vi "Save File DOE File Setup.vi"(0 "Filepath In":T10, 2 "Washer Controls In":T12={"Test Fixture Hardware"={"Power "={"Yokogawa"={"WT210"={"Sample Rate (1: 0.25s)"=1, "A Range (12: 20A)"=12, "V Range (6: 600V)"=4, "Power VISA Yokogawa WT210"="WT210"}, "WT500"={"Power VISA Yokogawa WT500"="WT500", "V Range (8: 1000V)"=0, "I Range (7: 40A)"=0, "Update Rate (3: 500ms)"=2}, "WT310_2"={"Sample Rate (1: 0.25s)"=1, "A Range (12: 20A)"=11, "V Range (6: 600V)"=4, "Power VISA Yokogawa WT310_2"="WT310_2"}, "WT310_3"={"Sample Rate (1: 0.25s)"=1, "A Range (12: 20A)"=11, "V Range (6: 600V)"=4, "Power VISA Yokogawa WT310_3"="WT310_3"}}, "Aplus"={"Aplus IP Address"="192.168.1.101", "Remote Port"=502, "Instrument"="APLUS", "Instr Driver Revision"="1.03.0053"}, "Power Limits"={"Crest Factor"={"Upper Limit"=1.49, "Lower Limit"=1.34}, "Harmonic Content"={"Uthd"=2.0}, "Voltage"={"% Error"=2.0}, "Stability"={"<1 Watt "={"Wattage"=1.0, "Slope (mW/H)"=10.0}, ">1 Watt"={"1%Power/Hour"=1.0}}}, "Nominal Voltage"=120, "Time Limit (s)"=10800.0, "Power Variation Limit (%)"=50.0, "Power Supply"={"Chroma 61605"="CHROMA", "Use Chroma?"=FALSE}}, "Weight Scale"={"Com Options"={"IND560Scale VISA"="IND560", "IP Address"="192.168.1.50", "Remote Port"=502, "Setra Scale VISA"="MW100", "GSE 350"="GSE350"}, "Select Scale"=""}, "Flow Rates"={"Laurel Cold IP Address"="", "Laurel Hot IP Address"="34972A_2", "Hot Water Laurel VISA"="LaurelMeter_Hot", "Cold Water Laurel VISA"="LaurelMeter_Cold", "Remote Port"=0, "Laurel Communication Type"="", "Meters To Collect (Hot Cold)"="", "HOT Laurel Reference"=refnum, "COLD Laurel Reference"=refnum}, "Analog Data"={"Agilent"={"Agilent 34972_1"="34972A_1", "Agilent 34972_2"="34972A_2", "Agilent 34972_3"="34972A_3", "Agilent 34972_4"="34972A_4", "Agilent 34972_5"="34972A_5", "Agilent 34972_6"="34972A_6", "Agilent Gain"=0.0, "TC Type (K,J,T)"="", "Instrument IDN?"="", "TC Channels-List"="", "Analog Channels-List"="", "Agilent Cluster Array"=[], "TC Channels-List 2"="", "Analog Channels-List 2"=""}, "Yokogawa"={"MW100"="MW100", "Intellifaucet"=FALSE}, "Select Analog"="", "TC Coefficients"={"TC Coefficients 1"=[], "TC Coefficients 2"=[], "TC Coefficients 3"=[], "TC Coefficients 4"=[], "TC Coefficients 5"=[], "TC Coefficients 6"=[], "TC Coefficients 7"=[]}, "NI Tasks (Dryer DOE)"=["TC Temps-Module 1", "TC Temps-Module 2", "TC Temps-Module 3", "TC Temps-Module 4", "TC Temps-Module 5", "Gas and Temp-Module 6", "AC_DC Events-Module 7"], "Laurel Analog"={"Laurel IP (Water Temp)"="", "Laurel IP (Pressure)"=""}}, "ITHX-Temp Humidity"={"IP Address 1"="", "Remote Port"=0, "IP Address 2"="", "IP Address 3"=""}, "Gas Meter COM Ports"={"Gas Meter 1"="COM3", "Gas Meter 2"="COM4", "Gas Meter 3"="COM5", "Gas Meter 4"="COM6", "Gas Meter 5"="COM7", "Gas Meter 6"="COM8"}, "Barometric Pressure"={"HEISE 901A"="HEISE", "Use Barometer?"=FALSE}}, "GEA2"={"Address"=35, "Source"=228, "Viper/Hawk"=0}, "DOE Capacity Measurments"={"Weight 1"=35.0, "Model Number 1"="", "Temp 1"=0.0, "Serial Number 1"="", "Lab Number 1"="", "Lab Number 2"="", "Serial Number 2"="", "Temp 2"=0.0, "Model Number 2"="", "Weight 2"=0.0, "Lab Number 3"="", "Serial Number 3"="", "Temp 3"=0.0, "Model Number 3"="", "Weight 3"=0.0, "Lab Number 4"="", "Serial Number 4"="", "Temp 4"=0.0, "Model Number 4"="", "Weight 4"=0.0, "Capacity Measurment Output String"=[]}, "Initialize.Washer In"={"Appliance Details"={"FileVersionInfo"={"FileVersion"="", "ProductName"="", "InternalName"="", "CompanyName"="", "LegalCopyright"="", "FileDescription"=""}, "Dishwasher Info"={"Open Cup Weight (gm):"=0.0, "Auto Cup Weight (gm):"=0.0, "Detergent-Dish:"="", "Inlet Temperature-Dish:"="", "Cycle Mode-Dish:"="", "Unit Control-Dish:"="", "Manufacturer-Dish:"=""}, "Washer Info"={"Hot Water Temperature (Fahrenheit):"="", "Cold Water Temperature (Fahrenheit):"="", "Capacity (cu.ft):"=0.0, "Initial Cloth Weight:"=0.0, "Cloth Lot:"=60, "Model Family:"="", "Program Name:"="", "Cycle Selection:"="", "Wash Temperature:"="", "Rinse Temperature:"="", "Load Size:"=""}, "File Name Output Array"=[], "Calibration Output Array"=[], "Appliance Common"={"Engineer:"="", "Model Number:"="", "Serial Number:"="", "Comments:"="", "Station ID:"="", "Technician:"="", "TR Number:"="", "Lab ID:"="", "Voltage:"="", "Water Pressure (PSI):"="", "Test Date:"="", "Computer Name:"="", "IP Address:"="", "Ambient RH:"="", "Frequency:"="", "Build:"="", "Filename:"="", "Test Type:"="", "Load Run #:"=17, "Ambient Temperature (F):"="", "File Path:"=path "", "Cycles Per Year"=0}, "Water Heater"={"Heating Mode:"=""}, "Dryer"={"Heat Setting:"="", "Washer Water Temperature (60 ± 5°F):"=7, "Water Hardness (PPM):"=7, "Dryness Setting:"="", "Dryer Type:"="", "Exhaust:"="", "Drying Cycle:"="", "Load Type:"="", "Nominal Load Weight"="", "Dryer Initial IMC Data"={"Measured IMC (lbs)"=100.0, "Actual Initial RMC (%)"=7.0, "RMC (Desired %)"=5.0, "Bone Dry Wt(lbs)"=60.0, "Tolerance(%)"=0.0, "Actual Final RMC (%)"=7.0, "CEF (lbf/kWh)"=0.0, "Minimum Weight (lbf)"=0.0, "Average Weight (lbf)"=0.0, "Maximum Weight (lbf)"=0.0, "Measured IMC In Range?"=FALSE, "Moisture Reduction Factor"=55.5, "Field Use Factor"=1.04, "Empty Dryer Cold Weigth"=0.0, "Energy Standard"=enum."D2-Automatic Dryer", "Weight Cloth (lbs)"=0.0, "Relative Moisture Content (%)"=0.0, "Relative Moisture Content - Avg (%)"=0.0}}}, "Display Data (RLT)"={"Status Color"=0, "Serial Number Display"="", "Cycle Count Display"=0, "Station Label Display"="", "Current Run Start Time Display"=0.0, "Board ID Display"="", "RPM Display"=0, "Current Display"=0.0, "Current Path Display"=path "", "Saving Display"=FALSE, "Unit Type Display"=enum."", "Total Time On Display"=0.0, "UI Button"=FALSE}}} {"Initialize.Washer In"."Display Data (RLT)"."Current Display" format="%.2f"; "Initialize.Washer In"."Display Data (RLT)"."Cycle Count Display" format="%04d"; "Initialize.Washer In"."Appliance Details"."Dryer"."Dryer Initial IMC Data"."Maximum Weight (lbf)" format="%03_6g"; "Initialize.Washer In"."Appliance Details"."Dryer"."Dryer Initial IMC Data"."Average Weight (lbf)" format="%03_6g"; "Initialize.Washer In"."Appliance Details"."Dryer"."Dryer Initial IMC Data"."Minimum Weight (lbf)" format="%03_6g"; "Initialize.Washer In"."Appliance Details"."Dryer"."Dryer Initial IMC Data"."CEF (lbf/kWh)" format="%03_6g"; "Initialize.Washer In"."Appliance Details"."Dryer"."Dryer Initial IMC Data"."Actual Final RMC (%)" format="%03_6g"; "Initialize.Washer In"."Appliance Details"."Dryer"."Dryer Initial IMC Data"."Tolerance(%)" format="%0#_6g"; "Initialize.Washer In"."Appliance Details"."Dryer"."Dryer Initial IMC Data"."Bone Dry Wt(lbs)" format="%03_6g"; "Initialize.Washer In"."Appliance Details"."Dryer"."Dryer Initial IMC Data"."RMC (Desired %)" format="%0#_6g"; "Initialize.Washer In"."Appliance Details"."Dryer"."Dryer Initial IMC Data"."Actual Initial RMC (%)" format="%03_6g"; "Initialize.Washer In"."Appliance Details"."Dryer"."Dryer Initial IMC Data"."Measured IMC (lbs)" format="%0#_6g"; "GEA2"."Address" format="%x"; "GEA2"."Source" format="%x"; "GEA2"."Viper/Hawk" items=["Viper", "Hawk"]; "Test Fixture Hardware"."Power"."Yokogawa"."WT310_3"."V Range (6: 600V)" items=["Auto", "15V", "30V", "60V", "150V", "300V", "600V"]; "Test Fixture Hardware"."Power"."Yokogawa"."WT310_3"."A Range (12: 20A)" items=["Auto", "5mA", "10mA", "20mA", "50mA", "100mA", "200mA", "0.5A", "1A", "2A", "5A", "10A", "20A", "50mV", "100mV", "200mV", "2.5V", "5V", "10V"]; "Test Fixture Hardware"."Power"."Yokogawa"."WT310_3"."Sample Rate (1: 0.25s)" items=["0.1s", "0.25s", "0.5s", "1s", "2s", "5s"]; "Test Fixture Hardware"."Power"."Yokogawa"."WT310_2"."V Range (6: 600V)" items=["Auto", "15V", "30V", "60V", "150V", "300V", "600V"]; "Test Fixture Hardware"."Power"."Yokogawa"."WT310_2"."A Range (12: 20A)" items=["Auto", "5mA", "10mA", "20mA", "50mA", "100mA", "200mA", "0.5A", "1A", "2A", "5A", "10A", "20A", "50mV", "100mV", "200mV", "2.5V", "5V", "10V"]; "Test Fixture Hardware"."Power"."Yokogawa"."WT310_2"."Sample Rate (1: 0.25s)" items=["0.1s", "0.25s", "0.5s", "1s", "2s", "5s"]; "Test Fixture Hardware"."Power"."Yokogawa"."WT500"."Update Rate (3: 500ms)" items=["-", "100ms", "200ms", "500ms", "1s", "2s", "5s"]; "Test Fixture Hardware"."Power"."Yokogawa"."WT500"."I Range (7: 40A)" items=["AUTO", "500 mA", "1 A", "2 A", "5 A", "10 A", "20 A", "40 A", "S-AUTO", "50 mV", "100 mV", "200 mV", "500 mV", "1 V", "2 V", "5 V", "10 V", "250 mA", "500 mA", "1 A", "2.5 A", "5 A", "10 A", "20 A", "25 mV", "50 mV", "100 mV", "250 mV", "500 mV", "1 V", "2.5 V", "5 V"]; "Test Fixture Hardware"."Power"."Yokogawa"."WT500"."V Range (8: 1000V)" items=["AUTO", "15", "30", "60", "100", "150", "300", "600", "1000", "7.5", "15", "30", "50", "75", "150", "300", "500"]; "Test Fixture Hardware"."Power"."Yokogawa"."WT210"."V Range (6: 600V)" items=["Auto", "15V", "30V", "60V", "150V", "300V", "600V"]; "Test Fixture Hardware"."Power"."Yokogawa"."WT210"."A Range (12: 20A)" items=["Auto", "5mA", "10mA", "20mA", "50mA", "100mA", "200mA", "0.5A", "1A", "2A", "5A", "10A", "20A", "50mV", "100mV", "200mV", "2.5V", "5V", "10V"]; "Test Fixture Hardware"."Power"."Yokogawa"."WT210"."Sample Rate (1: 0.25s)" items=["0.1s", "0.25s", "0.5s", "1s", "2s", "5s"]}, 3 "Station ID:":string(combo), 5 "error in (no error)":errorcluster, 6 "Config State":T8, 8 "LV Program":T9=enum."DOE Stand") -> (14 "Washer Controls Out":T12={"Test Fixture Hardware"={"Power "={"Yokogawa"={"WT210"={"Sample Rate (1: 0.25s)"=1, "A Range (12: 20A)"=12, "V Range (6: 600V)"=4, "Power VISA Yokogawa WT210"="WT210"}, "WT500"={"Power VISA Yokogawa WT500"="WT500", "V Range (8: 1000V)"=0, "I Range (7: 40A)"=0, "Update Rate (3: 500ms)"=2}, "WT310_2"={"Sample Rate (1: 0.25s)"=1, "A Range (12: 20A)"=11, "V Range (6: 600V)"=4, "Power VISA Yokogawa WT310_2"="WT310_2"}, "WT310_3"={"Sample Rate (1: 0.25s)"=1, "A Range (12: 20A)"=11, "V Range (6: 600V)"=4, "Power VISA Yokogawa WT310_3"="WT310_3"}}, "Aplus"={"Aplus IP Address"="192.168.1.101", "Remote Port"=502, "Instrument"="APLUS", "Instr Driver Revision"="1.03.0053"}, "Power Limits"={"Crest Factor"={"Upper Limit"=1.49, "Lower Limit"=1.34}, "Harmonic Content"={"Uthd"=2.0}, "Voltage"={"% Error"=2.0}, "Stability"={"<1 Watt "={"Wattage"=1.0, "Slope (mW/H)"=10.0}, ">1 Watt"={"1%Power/Hour"=1.0}}}, "Nominal Voltage"=120, "Time Limit (s)"=10800.0, "Power Variation Limit (%)"=50.0, "Power Supply"={"Chroma 61605"="CHROMA", "Use Chroma?"=FALSE}}, "Weight Scale"={"Com Options"={"IND560Scale VISA"="IND560", "IP Address"="192.168.1.50", "Remote Port"=502, "Setra Scale VISA"="SETRA", "GSE 350"="GSE350"}, "Select Scale"=""}, "Flow Rates"={"Laurel Cold IP Address"="", "Laurel Hot IP Address"="", "Hot Water Laurel VISA"="34972A_3", "Cold Water Laurel VISA"="MW100", "Remote Port"=0, "Laurel Communication Type"="", "Meters To Collect (Hot Cold)"="", "HOT Laurel Reference"=refnum, "COLD Laurel Reference"=refnum}, "Analog Data"={"Agilent"={"Agilent 34972_1"="34972A_1", "Agilent 34972_2"="34972A_2", "Agilent 34972_3"="34972A_3", "Agilent 34972_4"="34972A_3", "Agilent 34972_5"="34972A_3", "Agilent 34972_6"="34972A_3", "Agilent Gain"=0.0, "TC Type (K,J,T)"="", "Instrument IDN?"="", "TC Channels-List"="", "Analog Channels-List"="", "Agilent Cluster Array"=[], "TC Channels-List 2"="", "Analog Channels-List 2"=""}, "Yokogawa"={"MW100"="MW100", "Intellifaucet"=FALSE}, "Select Analog"="", "TC Coefficients"={"TC Coefficients 1"=[], "TC Coefficients 2"=[], "TC Coefficients 3"=[], "TC Coefficients 4"=[], "TC Coefficients 5"=[], "TC Coefficients 6"=[], "TC Coefficients 7"=[]}, "NI Tasks (Dryer DOE)"=["TC Temps-Module 1", "TC Temps-Module 2", "TC Temps-Module 3", "TC Temps-Module 4", "TC Temps-Module 5", "Gas and Temp-Module 6", "AC_DC Events-Module 7"], "Laurel Analog"={"Laurel IP (Water Temp)"="", "Laurel IP (Pressure)"=""}}, "ITHX-Temp Humidity"={"IP Address 1"="", "Remote Port"=0, "IP Address 2"="", "IP Address 3"=""}, "Gas Meter COM Ports"={"Gas Meter 1"="COM3", "Gas Meter 2"="COM4", "Gas Meter 3"="COM5", "Gas Meter 4"="COM6", "Gas Meter 5"="COM7", "Gas Meter 6"="COM8"}, "Barometric Pressure"={"HEISE 901A"="HEISE", "Use Barometer?"=FALSE}}, "GEA2"={"Address"=35, "Source"=228, "Viper/Hawk"=0}, "DOE Capacity Measurments"={"Weight 1"=35.0, "Model Number 1"="", "Temp 1"=0.0, "Serial Number 1"="", "Lab Number 1"="", "Lab Number 2"="", "Serial Number 2"="", "Temp 2"=0.0, "Model Number 2"="", "Weight 2"=0.0, "Lab Number 3"="", "Serial Number 3"="", "Temp 3"=0.0, "Model Number 3"="", "Weight 3"=0.0, "Lab Number 4"="", "Serial Number 4"="", "Temp 4"=0.0, "Model Number 4"="", "Weight 4"=0.0, "Capacity Measurment Output String"=[]}, "Initialize.Washer In"={"Appliance Details"={"FileVersionInfo"={"FileVersion"="", "ProductName"="", "InternalName"="", "CompanyName"="", "LegalCopyright"="", "FileDescription"=""}, "Dishwasher Info"={"Open Cup Weight (gm):"=0.0, "Auto Cup Weight (gm):"=0.0, "Detergent-Dish:"="", "Inlet Temperature-Dish:"="", "Cycle Mode-Dish:"="", "Unit Control-Dish:"="", "Manufacturer-Dish:"=""}, "Washer Info"={"Hot Water Temperature (Fahrenheit):"="", "Cold Water Temperature (Fahrenheit):"="", "Capacity (cu.ft):"=0.0, "Initial Cloth Weight:"=0.0, "Cloth Lot:"=60, "Model Family:"="", "Program Name:"="", "Cycle Selection:"="", "Wash Temperature:"="", "Rinse Temperature:"="", "Load Size:"=""}, "File Name Output Array"=[], "Calibration Output Array"=[], "Appliance Common"={"Engineer:"="", "Model Number:"="", "Serial Number:"="", "Comments:"="", "Station ID:"="", "Technician:"="", "TR Number:"="", "Lab ID:"="", "Voltage:"="", "Water Pressure (PSI):"="", "Test Date:"="", "Computer Name:"="", "IP Address:"="", "Ambient RH:"="", "Frequency:"="", "Build:"="", "Filename:"="", "Test Type:"="", "Load Run #:"=17, "Ambient Temperature (F):"="", "File Path:"=path "", "Cycles Per Year"=0}, "Water Heater"={"Heating Mode:"=""}, "Dryer"={"Heat Setting:"="", "Washer Water Temperature (60 ± 5°F):"=7, "Water Hardness (PPM):"=7, "Dryness Setting:"="", "Dryer Type:"="", "Exhaust:"="", "Drying Cycle:"="", "Load Type:"="", "Nominal Load Weight"="", "Dryer Initial IMC Data"={"Measured IMC (lbs)"=100.0, "Actual Initial RMC (%)"=7.0, "RMC (Desired %)"=5.0, "Bone Dry Wt(lbs)"=60.0, "Tolerance(%)"=0.0, "Actual Final RMC (%)"=7.0, "CEF (lbf/kWh)"=0.0, "Minimum Weight (lbf)"=0.0, "Average Weight (lbf)"=0.0, "Maximum Weight (lbf)"=0.0, "Measured IMC In Range?"=FALSE, "Moisture Reduction Factor"=55.5, "Field Use Factor"=1.04, "Empty Dryer Cold Weigth"=0.0, "Energy Standard"=enum."D2-Automatic Dryer", "Weight Cloth (lbs)"=0.0, "Relative Moisture Content (%)"=0.0, "Relative Moisture Content - Avg (%)"=0.0}}}, "Display Data (RLT)"={"Status Color"=0, "Serial Number Display"="", "Cycle Count Display"=0, "Station Label Display"="", "Current Run Start Time Display"=0.0, "Board ID Display"="", "RPM Display"=0, "Current Display"=0.0, "Current Path Display"=path "", "Saving Display"=FALSE, "Unit Type Display"=enum."", "Total Time On Display"=0.0, "UI Button"=FALSE}}} {"Initialize.Washer In"."Display Data (RLT)"."Current Display" format="%.2f"; "Initialize.Washer In"."Display Data (RLT)"."Cycle Count Display" format="%04d"; "Initialize.Washer In"."Appliance Details"."Dryer"."Dryer Initial IMC Data"."Maximum Weight (lbf)" format="%03_6g"; "Initialize.Washer In"."Appliance Details"."Dryer"."Dryer Initial IMC Data"."Average Weight (lbf)" format="%03_6g"; "Initialize.Washer In"."Appliance Details"."Dryer"."Dryer Initial IMC Data"."Minimum Weight (lbf)" format="%03_6g"; "Initialize.Washer In"."Appliance Details"."Dryer"."Dryer Initial IMC Data"."CEF (lbf/kWh)" format="%03_6g"; "Initialize.Washer In"."Appliance Details"."Dryer"."Dryer Initial IMC Data"."Actual Final RMC (%)" format="%03_6g"; "Initialize.Washer In"."Appliance Details"."Dryer"."Dryer Initial IMC Data"."Tolerance(%)" format="%0#_6g"; "Initialize.Washer In"."Appliance Details"."Dryer"."Dryer Initial IMC Data"."Bone Dry Wt(lbs)" format="%03_6g"; "Initialize.Washer In"."Appliance Details"."Dryer"."Dryer Initial IMC Data"."RMC (Desired %)" format="%0#_6g"; "Initialize.Washer In"."Appliance Details"."Dryer"."Dryer Initial IMC Data"."Actual Initial RMC (%)" format="%03_6g"; "Initialize.Washer In"."Appliance Details"."Dryer"."Dryer Initial IMC Data"."Measured IMC (lbs)" format="%0#_6g"; "GEA2"."Address" format="%x"; "GEA2"."Source" format="%x"; "GEA2"."Viper/Hawk" items=["Viper", "Hawk"]; "Test Fixture Hardware"."Power"."Yokogawa"."WT310_3"."V Range (6: 600V)" items=["Auto", "15V", "30V", "60V", "150V", "300V", "600V"]; "Test Fixture Hardware"."Power"."Yokogawa"."WT310_3"."A Range (12: 20A)" items=["Auto", "5mA", "10mA", "20mA", "50mA", "100mA", "200mA", "0.5A", "1A", "2A", "5A", "10A", "20A", "50mV", "100mV", "200mV", "2.5V", "5V", "10V"]; "Test Fixture Hardware"."Power"."Yokogawa"."WT310_3"."Sample Rate (1: 0.25s)" items=["0.1s", "0.25s", "0.5s", "1s", "2s", "5s"]; "Test Fixture Hardware"."Power"."Yokogawa"."WT310_2"."V Range (6: 600V)" items=["Auto", "15V", "30V", "60V", "150V", "300V", "600V"]; "Test Fixture Hardware"."Power"."Yokogawa"."WT310_2"."A Range (12: 20A)" items=["Auto", "5mA", "10mA", "20mA", "50mA", "100mA", "200mA", "0.5A", "1A", "2A", "5A", "10A", "20A", "50mV", "100mV", "200mV", "2.5V", "5V", "10V"]; "Test Fixture Hardware"."Power"."Yokogawa"."WT310_2"."Sample Rate (1: 0.25s)" items=["0.1s", "0.25s", "0.5s", "1s", "2s", "5s"]; "Test Fixture Hardware"."Power"."Yokogawa"."WT500"."Update Rate (3: 500ms)" items=["-", "100ms", "200ms", "500ms", "1s", "2s", "5s"]; "Test Fixture Hardware"."Power"."Yokogawa"."WT500"."I Range (7: 40A)" items=["AUTO", "500 mA", "1 A", "2 A", "5 A", "10 A", "20 A", "40 A", "S-AUTO", "50 mV", "100 mV", "200 mV", "500 mV", "1 V", "2 V", "5 V", "10 V", "250 mA", "500 mA", "1 A", "2.5 A", "5 A", "10 A", "20 A", "25 mV", "50 mV", "100 mV", "250 mV", "500 mV", "1 V", "2.5 V", "5 V"]; "Test Fixture Hardware"."Power"."Yokogawa"."WT500"."V Range (8: 1000V)" items=["AUTO", "15", "30", "60", "100", "150", "300", "600", "1000", "7.5", "15", "30", "50", "75", "150", "300", "500"]; "Test Fixture Hardware"."Power"."Yokogawa"."WT210"."V Range (6: 600V)" items=["Auto", "15V", "30V", "60V", "150V", "300V", "600V"]; "Test Fixture Hardware"."Power"."Yokogawa"."WT210"."A Range (12: 20A)" items=["Auto", "5mA", "10mA", "20mA", "50mA", "100mA", "200mA", "0.5A", "1A", "2A", "5A", "10A", "20A", "50mV", "100mV", "200mV", "2.5V", "5V", "10V"]; "Test Fixture Hardware"."Power"."Yokogawa"."WT210"."Sample Rate (1: 0.25s)" items=["0.1s", "0.25s", "0.5s", "1s", "2s", "5s"]}, 16 "Filepath Out":T10, 19 "error out":errorcluster)   [LabVIEW 2016, in "File Setup.lvlib"]
uses:
  File Setup.lvlib
  Custom Pallet Controls/Custom Pallet String.ctl
  Custom Pallet Controls/Custom Pallet Forward.ctl
  Type Definition/Save File DOE LabView Program.ctl
  Type Definition/Save File DOE File Path Control.ctl
  Type Definition/Save File DOE Data Save Filepaths.ctl
  Type Definition/Save File DOE Configuration State.ctl
  Type Definition/Save File HEWH Heating Control Mode.ctl
  Washer DOE/Type Definitions/DOE Main Control.ctl
  Washer DOE/Type Definitions/DOE Test Fixture Hardware.ctl
  Type Definitions/UTILITY Power Inputs Control.ctl
  Drivers/IND560 Scale Monitor/Type Definitions/IND560 Configuration.ctl
  Hybrid Water Heater/Type Definitions/HEWH Agilent Cluster.ctl
  Type Definitions/UTILITY TC Coefficients.ctl
  Drivers/Omega FMA-1600A Series Gas Flow Meter/Type Definitions/FMA1600A COM Ports.ctl
  Washer DOE/Configuration/GEA2.ctl
  Washer DOE/Type Definitions/DOE Capacity Measurments.ctl
  Public/Type Definitions/Save File Washer.ctl
  Type Definition/Save File DISH Dishwasher Details.ctl
  <vilib>/Platform/fileVersionInfo.llb/FileVersionInformation.ctl
  Washer DOE/Type Definitions/DOE Appliance Common.ctl
  Type Definition/DPT IMC Data.ctl
  Washer DOE/Type Definitions/DOE Dryer Standard.ctl
  Public/Type Definitions/Save File Appliance Display.ctl
  Public/Type Definitions/Save File Unit Type.ctl
  Type Definition/Save File Drop Down Controls.ctl
  <vilib>/Utility/file.llb/Write To Spreadsheet File (string).vi
  Save File.lvlib
panel:
  in  "Read Previous":bool
  in  "Comments:":string
  in  "Program Tab":T1(tab)
  in  "Remove Button 23":bool
  in  "Add Button 23":bool
  in  "Ambient Temperature (F):":string(combo)
  in  "Remove Button 17":bool
  in  "Add Button 17":bool
  in  "Lab ID:":string(combo)
  in  "Remove Button 1":bool
  in  "Add Button 1":bool
  in  "Remove Button 2":bool
  in  "Add Button 2":bool
  in  "Technician:":string(combo)
  in  "Remove Button 3":bool
  in  "Add Button 3":bool
  in  "Water Pressure (PSI):":string(combo)
  in  "Remove Button 4":bool
  in  "Add Button 4":bool
  in  "Ambient RH:":string(combo)
  in  "Remove Button 5":bool
  in  "Add Button 5":bool
  in  "Supply Voltage:":string(combo)
  in  "Remove Button 6":bool
  in  "Add Button 6":bool
  in  "Frequency:":string(combo)
  in  "Remove Button 7":bool
  in  "Add Button 7":bool
  in  "Build:":string(combo)
  in  "TR Number:":string(combo)
  in  "Remove Button 16":bool
  in  "Add Button 16":bool
  in  "Remove Button 12":bool
  in  "Add Button 12":bool
  in  "Test Type:":string(combo)
  in  "Load Run #:":i32
  in  "Model:":T2
  in  "Serial Number:":T2
  in  "Engineer:":T2
  in  "Cycles Per Year":u32=283
  in  "Remove Button 21":bool
  in  "Add Button 21":bool
  in  "Cycle Selection":string(combo)
  in  "Remove Button 18":bool
  in  "Add Button 18":bool
  in  "Wash Temperature":string(combo)
  in  "Remove Button 19":bool
  in  "Add Button 19":bool
  in  "Rinse Temperature":string(combo)
  in  "Remove Button 20":bool
  in  "Add Button 20":bool
  in  "Load Size":string(combo)
  in  "Remove Button 9":bool
  in  "Add Button 9":bool
  in  "Cold Water Temperature (Fahrenheit)":string(combo)
  in  "Program Name":string(combo)
  in  "Model Family":string(combo)
  in  "Cloth Lot:":i32
  in  "Initial Cloth Weight:":dbl
  in  "Capacity (cu.ft)":dbl
  in  "Hot Water Temperature (Fahrenheit)":string(combo)
  in  "Remove Button 8":bool
  in  "Add Button 8":bool
  in  "Unit Type Display":T3
  in  "Remove Button 15":bool
  in  "Add Button 15":bool
  in  "Detergent-Dish:":string(combo)
  in  "Remove Button 14":bool
  in  "Add Button 14":bool
  in  "Inlet Temperature-Dish:":string(combo)
  in  "Remove Button 13":bool
  in  "Add Button 13":bool
  in  "Cycle Mode-Dish:":string(combo)
  in  "Remove Button 11":bool
  in  "Add Button 11":bool
  in  "Unit Control-Dish:":string(combo)
  in  "Manufacturer-Dish:":string(combo)
  in  "Remove Button 10":bool
  in  "Add Button 10":bool
  in  "Auto Cup Weight (gm):":dbl
  in  "Open Cup Weight (gm):":dbl
  in  "Heating Mode":T4
  in  "Remove Button 22":bool
  in  "Add Button 22":bool
  in  "Energy Standard":T5
  in  "Field Use Factor":dbl
  in  "Moisture Reduction Factor":dbl=55.5
  in  "Get Data":bool
  out "In Range?":string
  in  "Measured Weight (lbf)":dbl format="%#_5g"
  out "Measured Conent (%)":dbl format="%#_5g"
  out "Maximum Weight (lbf)":dbl format="%#_5g"
  out "Average Weight (lbf)":dbl format="%#_5g"
  out "Minimum Weight (lbf)":dbl format="%#_5g"
  in  "Tolerance (%)":dbl=0.33 format="%#_5g"
  in  "Relative Moisture (%)":dbl min=0.0 max=100.0 format="%#_5g"
  in  "Bone Dry Weight (lbf)":dbl min=0.0 max=100.0 format="%#_5g"
  in  "Remove Button 30":bool
  in  "Remove Button 29":bool
  in  "Remove Button 28":bool
  in  "Remove Button 27":bool
  in  "Remove Button 26":bool
  in  "Remove Button 25":bool
  in  "Remove Button 24":bool
  in  "Add Button 30":bool
  in  "Add Button 29":bool
  in  "Add Button 28":bool
  in  "Add Button 27":bool
  in  "Add Button 26":bool
  in  "Add Button 25":bool
  in  "Add Button 24":bool
  in  "Load Type:":string(combo)
  in  "Nominal Load Weight (lbs):":string(combo)
  in  "Dryness Setting:":string(combo)
  in  "Heat Setting:":string(combo)
  in  "Get Weigth":bool
  in  "Cold Dryer Weigth":dbl
  in  "Drying Cycle:":string(combo)
  in  "Exhaust:":string(combo)
  in  "Water Hardness (PPM):":u16=17
  in  "Washer Water Temperature (60 ± 5°F):":u16=60
  in  "Dryer Type:":string(combo)
  in  "Save As Default":bool
  in  "Initialize Default":bool
  out "Description":string="File Name Setup"
  in  "OK":T6
  in  "Tab Control":T7(tab)
  out "Move Past Main Tab":bool
  out "Unhandled Error":errorcluster
  in  "Debug":bool
  out "States":string[](array[string])
  # "Field Use Factor = 1.04 (Automatic Termination)\nField Use Factor = 1.18 (Only Timer Dryers) \nD1 = [53.5/(Ww-Wd)] × Ett × field use"
  # "Field Use Factor = 1.18 (Only Timer Dryers) \nD2 = [55.5/(Ww- Wd)] × Et × field use (Timer Dryer Only)\nD2 = Et (Automatic Termination)"
  # "Target Values"
  # "Weight Range (lbf)"
  # "Actual Content"
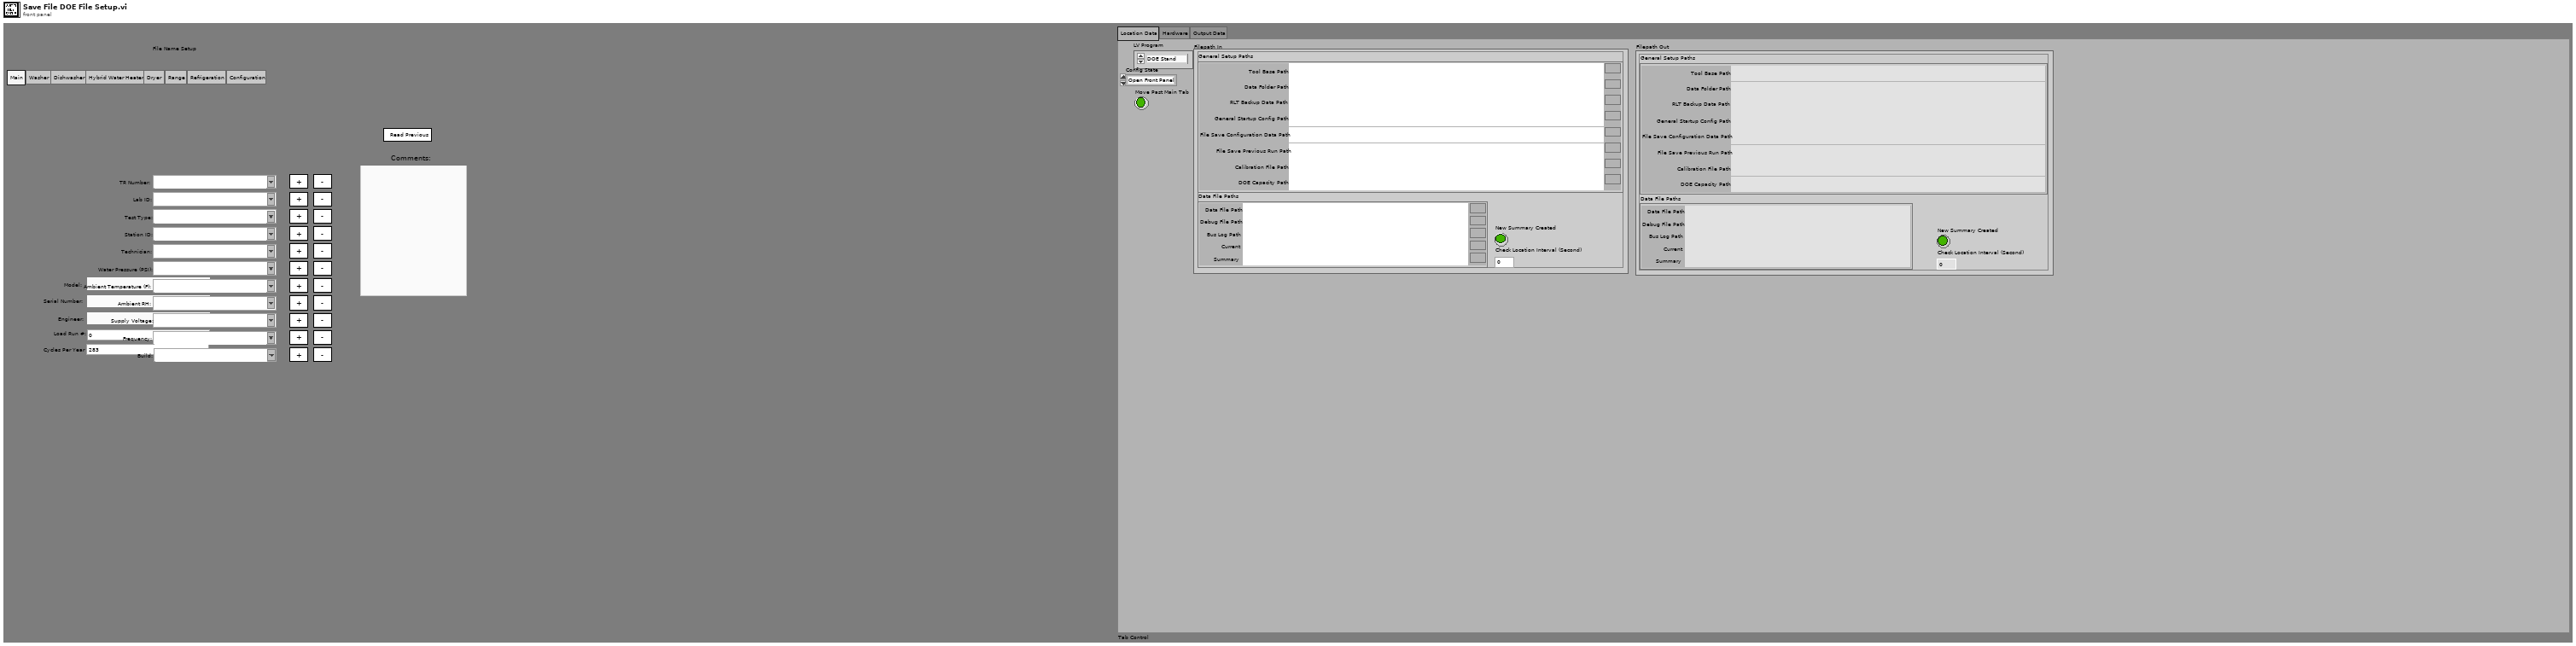
[diagram p1: front panel]
types:
  T1 = enum32{"Main", "Washer", "Dishwasher", "Hybrid Water Heater", "Dryer", "Range", "Refrigeration", "Configuration"}
  T2 = typedef "Custom Pallet String.ctl" = string
  T3 = typedef "Save File.lvlib/Save File Unit Type.ctl" = enum32{"", "Viper", "Hawk", "2015"}
  T4 = typedef "File Setup.lvlib/Save File HEWH Heating Control Mode.ctl" = string
  T5 = typedef "DOE Dryer Standard.ctl" = enum16{"D2-Automatic Dryer", "D2-Timer Dryer", "D1-Automatic Dryer", "D1-Timer Dryer", "Other"}
  T6 = typedef "Custom Pallet Forward.ctl" = bool
  T7 = enum32{"Location Data", "Hardware", "Output Data"}
  T8 = typedef "File Setup.lvlib/Save File DOE Configuration State.ctl" = enum16{"Open Front Panel", "Load Config"}
  T9 = typedef "File Setup.lvlib/Save File DOE LabView Program.ctl" = enum16{"No Name Found", "DOE Stand", "Dishwasher Kitchen", "Portable Stand", "HEWH", "Dryer", "Dryer WILT", "HCC", "PRAT", "HEWH RLT", "Refrigeration"}
  T10 = typedef "File Setup.lvlib/Save File DOE File Path Control.ctl" = cluster{"General Setup Paths":cluster{"Calibration File Path":path, "DOE Capacity Path":path, "Data Folder Path":path, "RLT Backup Data Path":path, "Tool Base Path":path, "General Startup Config Path":path, "File Save Previous Run Path":path, "File Save Configuration Data Path":path}, "Data File Paths":T11, "New Summary Created":bool, "Check Location Interval (Second)":i32}
  T11 = typedef "File Setup.lvlib/Save File DOE Data Save Filepaths.ctl" = cluster{"Data File Path":path, "Debug File Path":path, "Bus Log Path":path, "Current":path, "Summary":path}
  T12 = typedef "DOE Main Control.ctl" = cluster{"Test Fixture Hardware":T13, "GEA2":T19, "DOE Capacity Measurments":T20, "Initialize.Washer In":T21}
  T13 = typedef "DOE Test Fixture Hardware.ctl" = cluster{"Power ":T14, "Weight Scale":cluster{"Com Options":T15, "Select Scale":string}, "Flow Rates":cluster{"Laurel Cold IP Address":string, "Laurel Hot IP Address":string, "Hot Water Laurel VISA":refnum<visa-resource-name>, "Cold Water Laurel VISA":refnum<visa-resource-name>, "Remote Port":u16, "Laurel Communication Type":string, "Meters To Collect (Hot Cold)":string, "HOT Laurel Reference":refnum<k5>, "COLD Laurel Reference":refnum<k5>}, "Analog Data":cluster{"Agilent":cluster{"Agilent 34972_1":refnum<visa-resource-name>, "Agilent 34972_2":refnum<visa-resource-name>, "Agilent 34972_3":refnum<visa-resource-name>, "Agilent 34972_4":refnum<visa-resource-name>, "Agilent 34972_5":refnum<visa-resource-name>, "Agilent 34972_6":refnum<visa-resource-name>, "Agilent Gain":dbl, "TC Type (K,J,T)":string, "Instrument IDN?":string, "TC Channels-List":string, "Analog Channels-List":string, "Agilent Cluster Array":T16[], "TC Channels-List 2":string, "Analog Channels-List 2":string}, "Yokogawa":cluster{"MW100":refnum<visa-resource-name>, "Intellifaucet":bool}, "Select Analog":string, "TC Coefficients":T17, "NI Tasks (Dryer DOE)":refnum<k21>[], "Laurel Analog":cluster{"Laurel IP (Water Temp)":string, "Laurel IP (Pressure)":string}}, "ITHX-Temp Humidity":cluster{"IP Address 1":string, "Remote Port":u16, "IP Address 2":string, "IP Address 3":string}, "Gas Meter COM Ports":T18, "Barometric Pressure":cluster{"HEISE 901A":refnum<visa-resource-name>, "Use Barometer?":bool}}
  T14 = typedef "UTILITY Power Inputs Control.ctl" = cluster{"Yokogawa":cluster{"WT210":cluster{"Sample Rate (1: 0.25s)":i32, "A Range (12: 20A)":i32, "V Range (6: 600V)":i32, "Power VISA Yokogawa WT210":refnum<visa-resource-name>}, "WT500":cluster{"Power VISA Yokogawa WT500":refnum<visa-resource-name>, "V Range (8: 1000V)":i32, "I Range (7: 40A)":i32, "Update Rate (3: 500ms)":i32}, "WT310_2":cluster{"Sample Rate (1: 0.25s)":i32, "A Range (12: 20A)":i32, "V Range (6: 600V)":i32, "Power VISA Yokogawa WT310_2":refnum<visa-resource-name>}, "WT310_3":cluster{"Sample Rate (1: 0.25s)":i32, "A Range (12: 20A)":i32, "V Range (6: 600V)":i32, "Power VISA Yokogawa WT310_3":refnum<visa-resource-name>}}, "Aplus":cluster{"Aplus IP Address":string, "Remote Port":i32, "Instrument":string, "Instr Driver Revision":string}, "Power Limits":cluster{"Crest Factor":cluster{"Upper Limit":dbl, "Lower Limit":dbl}, "Harmonic Content":cluster{"Uthd":dbl}, "Voltage":cluster{"% Error":dbl}, "Stability":cluster{"<1 Watt ":cluster{"Wattage":dbl, "Slope (mW/H)":dbl}, ">1 Watt":cluster{"1%Power/Hour":dbl}}}, "Nominal Voltage":i32, "Time Limit (s)":dbl, "Power Variation Limit (%)":dbl, "Power Supply":cluster{"Chroma 61605":refnum<visa-resource-name>, "Use Chroma?":bool}}
  T15 = typedef "IND560 Configuration.ctl" = cluster{"IND560Scale VISA":refnum<visa-resource-name>, "IP Address":string, "Remote Port":u16, "Setra Scale VISA":refnum<visa-resource-name>, "GSE 350":refnum<visa-resource-name>}
  T16 = typedef "HEWH Agilent Cluster.ctl" = cluster{"Label":string, "Agilent Channel":string, "Panel ID":string, "Source":string, "Temperature":dbl}
  T17 = typedef "UTILITY TC Coefficients.ctl" = cluster{"TC Coefficients 1":dbl[], "TC Coefficients 2":dbl[], "TC Coefficients 3":dbl[], "TC Coefficients 4":dbl[], "TC Coefficients 5":dbl[], "TC Coefficients 6":dbl[], "TC Coefficients 7":dbl[]}
  T18 = typedef "FMA1600A COM Ports.ctl" = cluster{"Gas Meter 1":refnum<visa-resource-name>, "Gas Meter 2":refnum<visa-resource-name>, "Gas Meter 3":refnum<visa-resource-name>, "Gas Meter 4":refnum<visa-resource-name>, "Gas Meter 5":refnum<visa-resource-name>, "Gas Meter 6":refnum<visa-resource-name>}
  T19 = typedef "GEA2.ctl" = cluster{"Address":u8, "Source":u8, "Viper/Hawk":u8}
  T20 = typedef "DOE Capacity Measurments.ctl" = cluster{"Weight 1":dbl, "Model Number 1":string, "Temp 1":dbl, "Serial Number 1":string, "Lab Number 1":string, "Lab Number 2":string, "Serial Number 2":string, "Temp 2":dbl, "Model Number 2":string, "Weight 2":dbl, "Lab Number 3":string, "Serial Number 3":string, "Temp 3":dbl, "Model Number 3":string, "Weight 3":dbl, "Lab Number 4":string, "Serial Number 4":string, "Temp 4":dbl, "Model Number 4":string, "Weight 4":dbl, "Capacity Measurment Output String":string[][]}
  T21 = typedef "Save File.lvlib/Save File Washer.ctl" = cluster{"Appliance Details":T22, "Display Data (RLT)":T26}
  T22 = typedef "File Setup.lvlib/Save File DISH Dishwasher Details.ctl" = cluster{"FileVersionInfo":T23, "Dishwasher Info":cluster{"Open Cup Weight (gm):":dbl, "Auto Cup Weight (gm):":dbl, "Detergent-Dish:":string, "Inlet Temperature-Dish:":string, "Cycle Mode-Dish:":string, "Unit Control-Dish:":string, "Manufacturer-Dish:":string}, "Washer Info":cluster{"Hot Water Temperature (Fahrenheit):":string, "Cold Water Temperature (Fahrenheit):":string, "Capacity (cu.ft):":dbl, "Initial Cloth Weight:":dbl, "Cloth Lot:":i32, "Model Family:":string, "Program Name:":string, "Cycle Selection:":string, "Wash Temperature:":string, "Rinse Temperature:":string, "Load Size:":string}, "File Name Output Array":string[][], "Calibration Output Array":string[][], "Appliance Common":T24, "Water Heater":cluster{"Heating Mode:":string}, "Dryer":cluster{"Heat Setting:":T2, "Washer Water Temperature (60 ± 5°F):":u16, "Water Hardness (PPM):":u16, "Dryness Setting:":T2, "Dryer Type:":string, "Exhaust:":string, "Drying Cycle:":string, "Load Type:":string, "Nominal Load Weight":string, "Dryer Initial IMC Data":T25}}
  T23 = typedef "FileVersionInformation.ctl" = cluster{"FileVersion":string, "ProductName":string, "InternalName":string, "CompanyName":string, "LegalCopyright":string, "FileDescription":string}
  T24 = typedef "DOE Appliance Common.ctl" = cluster{"Engineer:":string, "Model Number:":string, "Serial Number:":string, "Comments:":string, "Station ID:":string, "Technician:":string, "TR Number:":string, "Lab ID:":string, "Voltage:":string, "Water Pressure (PSI):":string, "Test Date:":string, "Computer Name:":string, "IP Address:":string, "Ambient RH:":string, "Frequency:":string, "Build:":string, "Filename:":string, "Test Type:":string, "Load Run #:":i32, "Ambient Temperature (F):":string, "File Path:":path, "Cycles Per Year":u32}
  T25 = typedef "DPT IMC Data.ctl" = cluster{"Measured IMC (lbs)":dbl, "Actual Initial RMC (%)":dbl, "RMC (Desired %)":dbl, "Bone Dry Wt(lbs)":dbl, "Tolerance(%)":dbl, "Actual Final RMC (%)":dbl, "CEF (lbf/kWh)":dbl, "Minimum Weight (lbf)":dbl, "Average Weight (lbf)":dbl, "Maximum Weight (lbf)":dbl, "Measured IMC In Range?":bool, "Moisture Reduction Factor":dbl, "Field Use Factor":dbl, "Empty Dryer Cold Weigth":dbl, "Energy Standard":T5, "Weight Cloth (lbs)":dbl, "Relative Moisture Content (%)":dbl, "Relative Moisture Content - Avg (%)":dbl}
  T26 = typedef "Save File Appliance Display.ctl" = cluster{"Status Color":u32, "Serial Number Display":string, "Cycle Count Display":i32, "Station Label Display":string, "Current Run Start Time Display":dbl, "Board ID Display":string, "RPM Display":u32, "Current Display":dbl, "Current Path Display":path, "Saving Display":bool, "Unit Type Display":T3, "Total Time On Display":dbl, "UI Button":bool}
  T27 = enum16{"Load Standard", "Remove", "Add", "Update"}
  T28 = enum32{"invalid app kind", "Development System", "Run Time System", "Student Edition", "Embedded LabVIEW", "Evaluation", "Custom"}
  T29 = enum32{"Invalid", "Standard", "Closed", "Hidden", "Minimized", "Maximized"}
  T30 = typedef "File Setup.lvlib/Save File Drop Down Controls.ctl" = cluster{"Manufacturer-Dish (Array):":string[], "Unit Control-Dish (Array):":string[], "Test Type (Array):":string[], "Cycle Mode-Dish(Array): ":string[], "Inlet Temperature (F)-Dish (Array):":string[], "Detergent-Dish (Array):":string[], "Cycle Selection (Array):":string[], "Wash Temperature (Array):":string[], "Rinse Temperature (Array):":string[], "Load Size (Array):":string[], "Water Pressure (PSI) (Array) :":string[], "Ambient RH (Array):":string[], "Supply Voltage (Array):":string[], "Station ID (Array):":string[], "Lab ID (Array):":string[], "TR Number (Array):":string[], "Cold Water Temperature (Fahrenheit) (Array):":string[], "Technician (Array):":string[], "Frequency (Array):":string[], "Build (Array):":string[], "Hot Water Temperature (Fahrenheit) (Array):":string[], "Heating Mode (Array):":string[], "Ambient Temperature (F) (Array):":string[], "Dryer Type (Array):":string[], "Exhaust (Array):":string[], "Drying Cycle (Array):":string[], "Heat Setting (Array):":string[], "Dryness Setting (Array):":string[], "Nominal Load Weigth (lbs) (Array):":string[], "Load Type (Array):":string[]}
  T31 = cluster{"Core":cluster{"Current VI Reference":refnum<vi>, "Close Panel on Exit?":bool}, "Error Flag":bool, "Washer Controls In":T12, "LV Program":T9, "Filepath In":T10, "Drop Down Controls":T30}
  T32 = cluster{"Current VI Reference":refnum<vi>, "Close Panel on Exit?":bool}
  T33 = typedef "File Setup.lvlib/Save File DOE Configuration File.ctl" = cluster{"File Search":string[], "Model Details Header":string[], "Drop Down Controls":T30, "End of Cycle Commands":string[]}
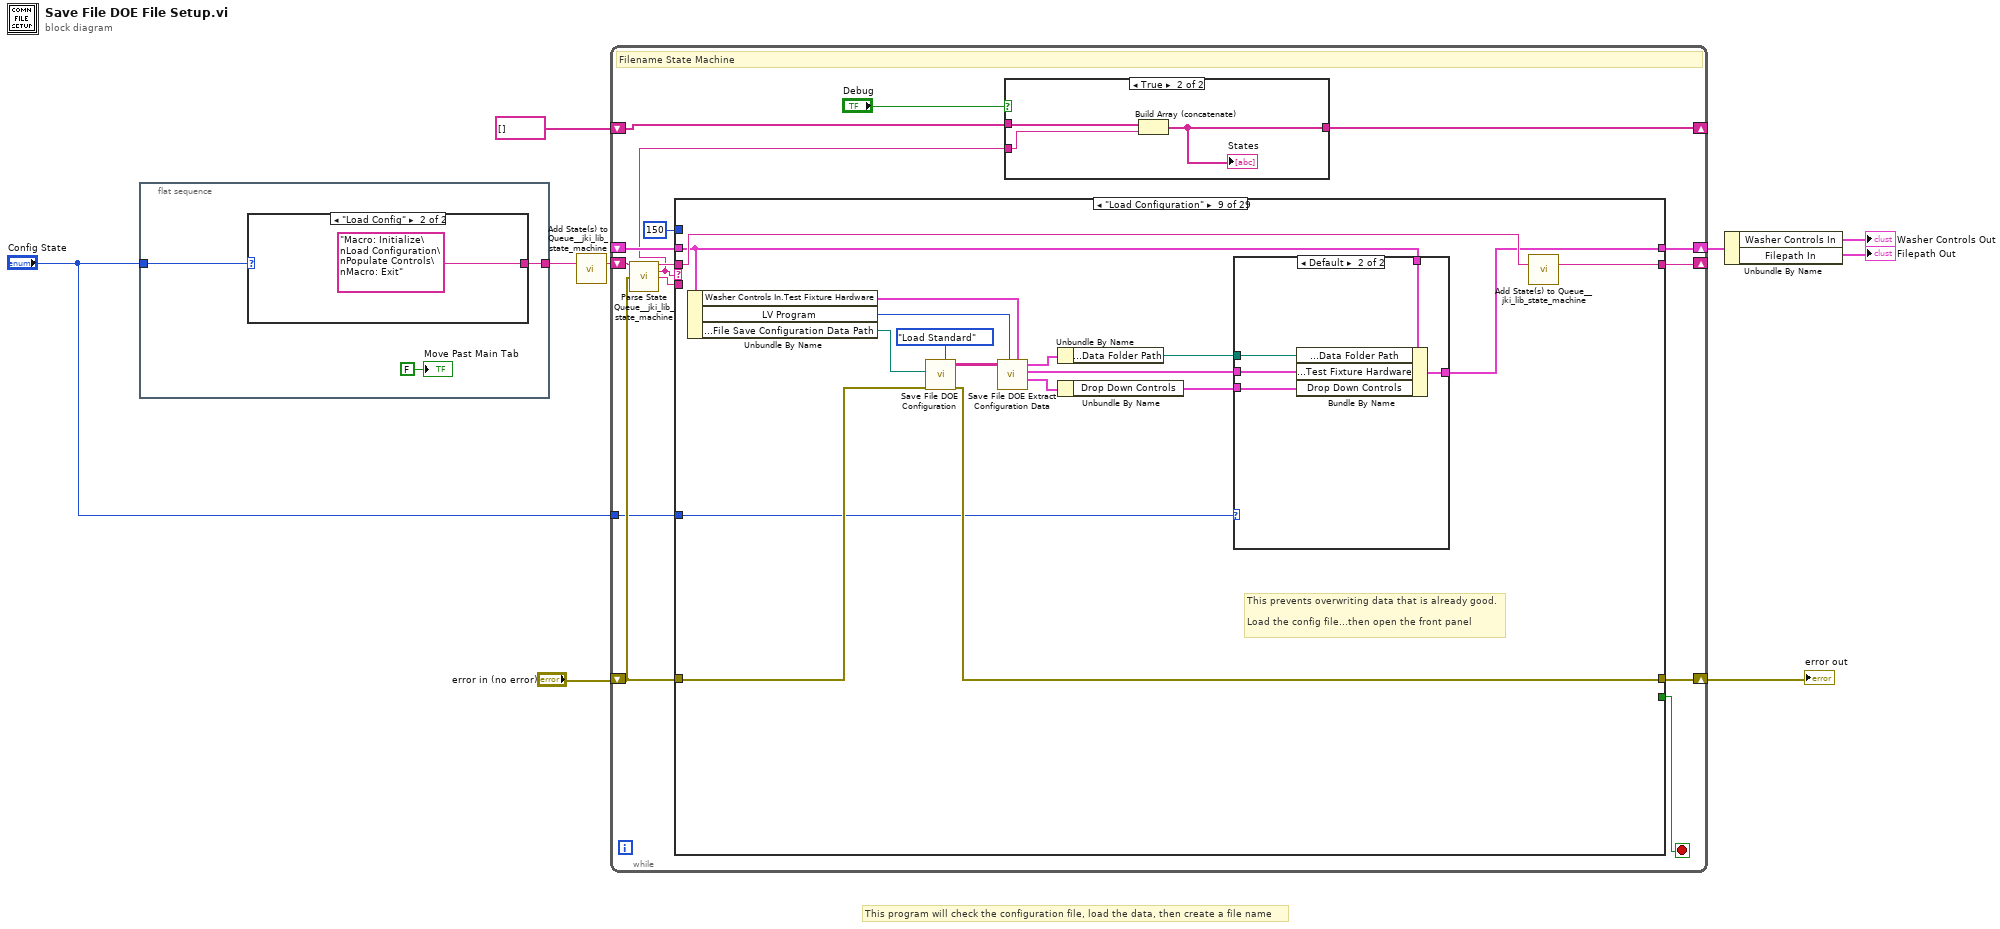
[diagram p0: block diagram]
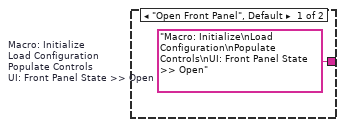
[diagram p2: hidden frame]
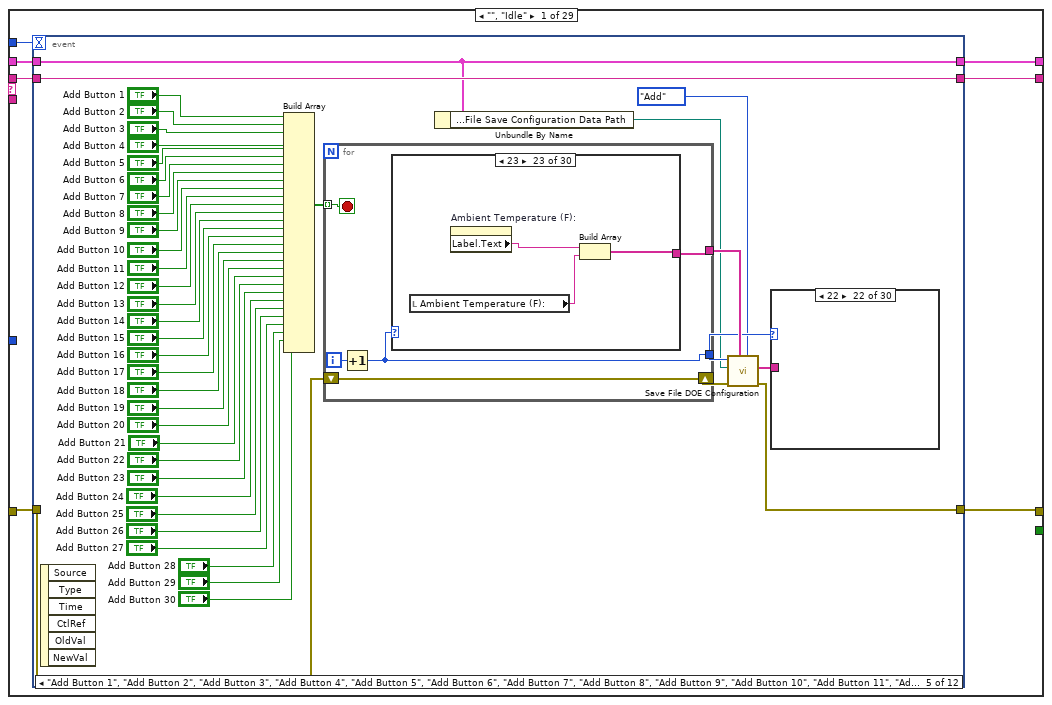
[diagram p4: hidden frame]
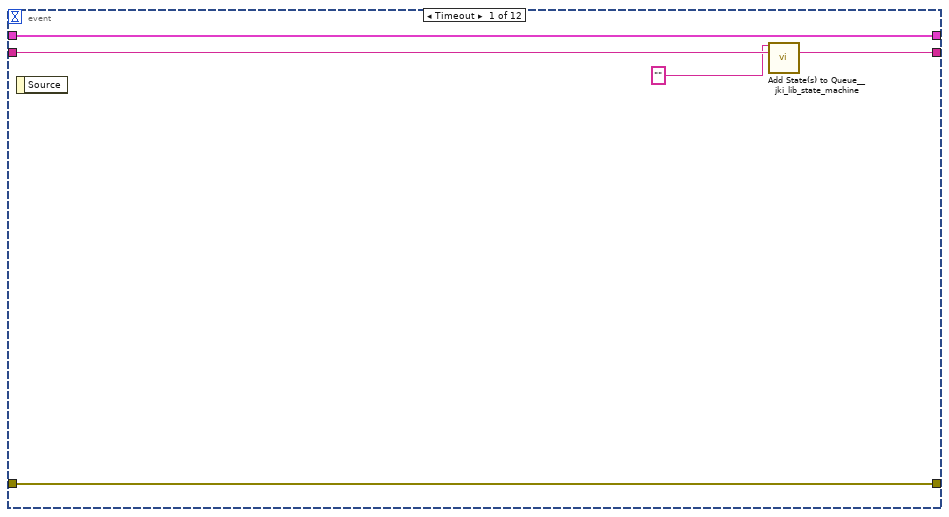
[diagram p5: hidden frame]
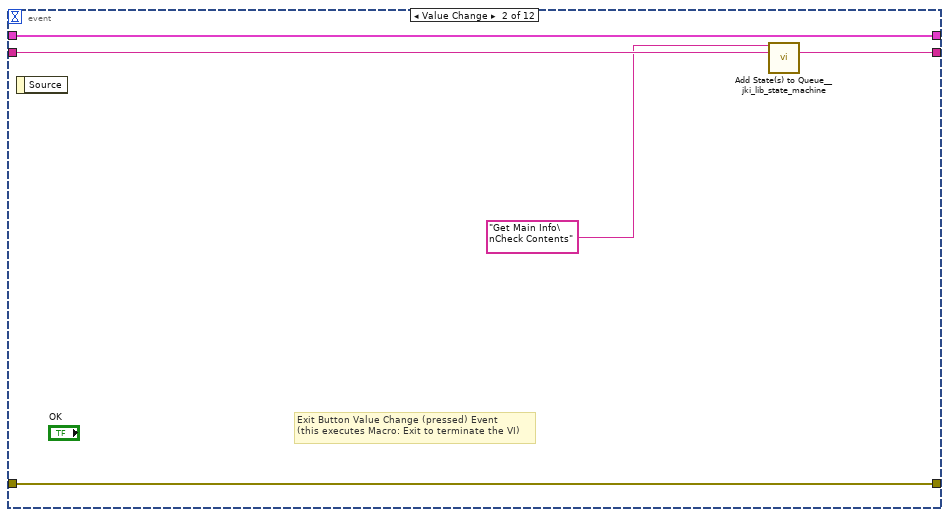
[diagram p6: hidden frame]
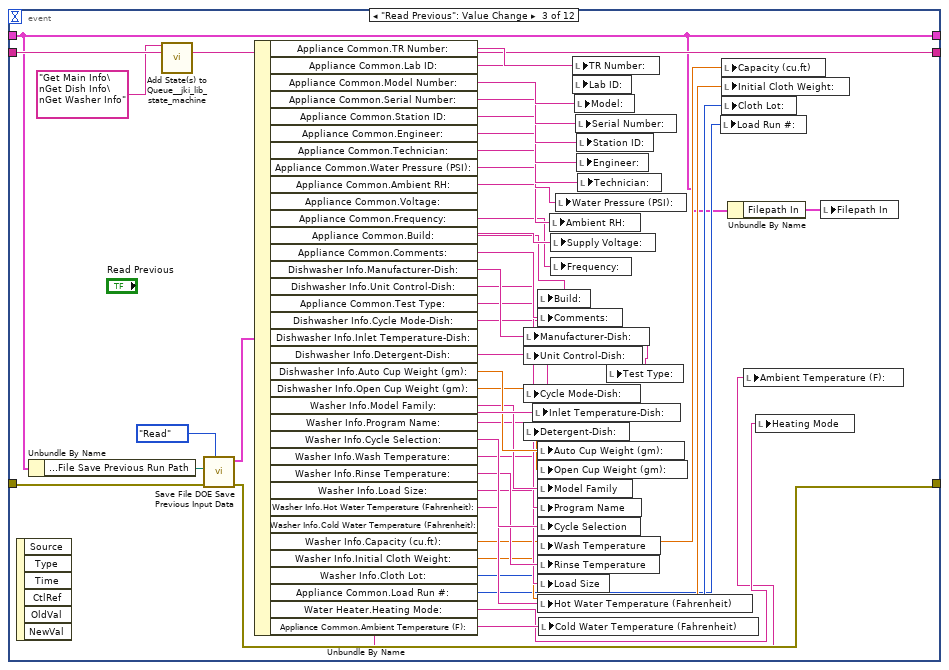
[diagram p7: hidden frame]
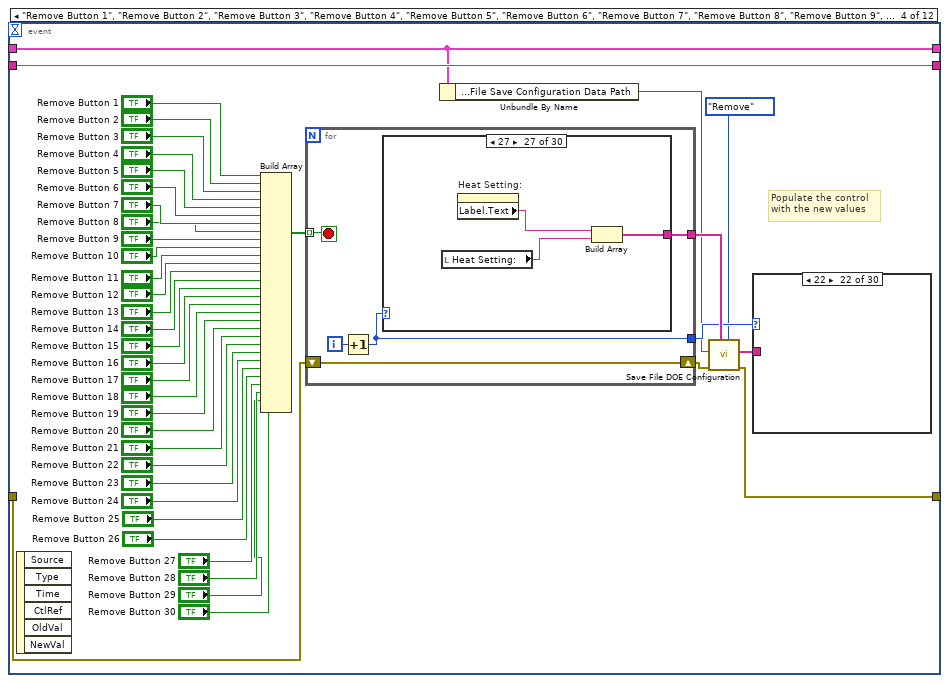
[diagram p8: hidden frame]
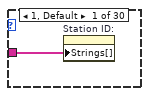
[diagram p9: hidden frame]
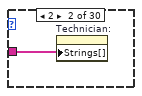
[diagram p10: hidden frame]
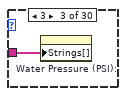
[diagram p11: hidden frame]
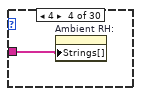
[diagram p12: hidden frame]
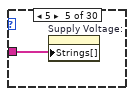
[diagram p13: hidden frame]
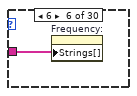
[diagram p14: hidden frame]
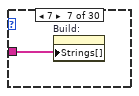
[diagram p15: hidden frame]
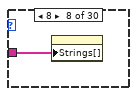
[diagram p16: hidden frame]
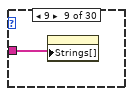
[diagram p17: hidden frame]
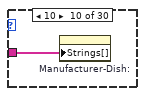
[diagram p18: hidden frame]
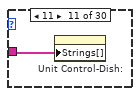
[diagram p19: hidden frame]
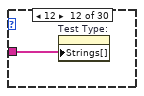
[diagram p20: hidden frame]
diagram:
  # "This program will check the configuration file, load the data, then create a file name"
  n1 = flat-sequence {
    tunnel: [w12] -> w5
    tunnel: "Config State" -> [w10]
    frame #0 {
      n2 = case shown="\"Load Config\"" w10 {
        tunnel: [w13 "Macro: Initialize\nLoad Configuration\nPopulate Controls\nMacro: Exit"] -> w12
        frame "Open Front Panel", Default {
          w13 = "Macro: Initialize\nLoad Configuration\nPopulate Controls\nUI: Front Panel State >> Open"  # Macro: Initialize Load Configuration Populate Controls UI: Front Panel State >> Open
        }
        frame "Load Config" {
        }
      }
      "Move Past Main Tab" <- FALSE ("Move Past Main Tab")
    }
  }
  n3 = call <vilib>:"Add State(s) to Queue__jki_lib_state_machine.vi"("State(s) in (\"\")"=w5) -> ("States Out"=w8:string)  [unwired: 14 in]
  n4 = while "Filename State Machine" {
    shift-right: [w23] -> w6
    shift-left: _ -> [w22]
    shift-right: [w26] -> w9
    shift-left: "error in (no error)" -> [w20]
    shift-right: [w25] -> _
    shift-left: w8 -> [w27]
    shift-right: [w18] -> _
    shift-left: string[] [] -> [w19]
    tunnel: "Config State" -> [w15]
    stop <- w24 stop-if-true
    # "Filename State Machine"
    n5 = call <vilib>:"Parse State Queue__jki_lib_state_machine.vi"("State Queue"=w27, "Error In (no error)"=w20) -> ("Remaining States"=w29:string, "Current State"=w17:string, "Arguments"=w28:string)  [unwired: 11 in]
    n6 = case shown="\"Load Configuration\"" w17 {
      selector: w17 -> [_ _ w534 _ _ _ _ _ _ _ _ _ _ _ _ _ _ _ _ _ _ _ _ _ _ _ _ _ _]
      tunnel: w29 -> [w40 w533 w538 w556 w564 w569 w573 w585 w602 w644 w650 w654 w672 w678 w689 w715 w722 w732 w736 w757 w779 w809 w839 w863 w889 w914 w933 w944 w954]
      tunnel: w28 -> [_ _ _ _ _ _ _ _ _ _ _ _ _ w673 w683 _ _ _ _ _ _ _ _ _ _ _ _ _ _]
      tunnel: w22 -> [w38 w530 w536 w548 w559 w567 w570 _ w597 w620 w645 w651 w664 w676 w685 w712 w719 w729 w733 w756 w775 w808 w838 w862 w888 w913 w930 w942 w948]
      tunnel: [w37 w531 w540 w545 errorcluster {"status"=FALSE, "code"=0, "source"=""} ("error out") w566 w571 w582 w600 w642 w646 w652 w663 w674 w686 w713 w720 w730 w734 w759 w777 w811 w841 w865 w891 w916 w923 w934 w945] -> w26
      tunnel: w20 -> [w36 w531 w539 w545 w561 w566 w571 w582 w599 w642 w647 w652 w657 w675 w687 w713 w720 w730 w734 w759 w777 w811 w841 w865 w891 w916 w924 w935 w946]
      tunnel: [w39 w532 w537 w555 w563 w568 w572 w584 w601 w643 w649 w653 w671 w677 w688 w714 w721 w731 w735 w760 w778 w812 w842 w866 w892 w917 w932 w943 w953] -> w25
      tunnel: [_ _ _ _ _ TRUE _ _ _ _ _ _ _ _ _ _ _ _ _ _ _ _ _ _ _ _ _ _ _] -> w24
      tunnel: [w35 w530 w536 w554 w558 w567 w570 w583 w592 w620 w645 w651 w656 w676 w685 w712 w719 w729 w733 w758 w774 w810 w840 w864 w890 w915 w931 w941 w948] -> w23
      tunnel: 150 ("Timeout") -> [w34 _ _ _ _ _ _ _ _ _ _ _ _ _ _ _ _ _ _ _ _ _ _ _ _ _ _ _ _]
      tunnel: w15 -> [_ _ _ _ _ _ _ _ w589 _ _ _ _ _ _ _ _ _ _ _ _ _ _ _ _ _ _ _ _]
      frame "", "Idle" {
        n7 = event shown="[4] \"Add Button 1\", \"Add Button 2\", \"Add Button 3\", \"Add Button 4\", \"Add Button 5\", \"Add Button 6\", \"Add Button 7\", \"Add Button 8\", \"Add Button 9\", \"Add Button 10\", \"Add Button 11\", \"Add Button 12\", \"Add Button 13\", \"Add Button 14\", \"Add Button 15\", \"Add Button 16\", \"Add Button 17\", \"Add Button 18\", \"Add Button 19\", \"Add Button 20\", \"Add Button 21\", \"Add Button 22\", \"Add Button 23\", \"Add Button 24\", \"Add Button 25\", \"Add Button 26\", \"Add Button 27\", \"Add Button 28\", \"Add Button 29\", \"Add Button 30\": Value Change" {
          selector: _ -> [_ _ _ _ _ _ _ _ _ _ _ _]
          dyn-events: _ -> [_ _ _ _ _ _ _ _ _ _ _ _]
          timeout: w34 -> [_ _ _ _ _ _ _ _ _ _ _ _]
          tunnel: w40 -> [w45 w50 w57 w136 w286 w433 w438 w461 w468 w491 w506 w529]
          tunnel: [w44 w49 w56 w136 w286 w432 w438 w461 w468 w491 w507 w528] -> w39
          tunnel: w38 -> [w41 w47 w51 w106 w271 w434 w437 w459 w470 w485 w505 w526]
          tunnel: [w43 w48 w94 w120 w277 w428 w439 w445 w466 w490 w508 w527] -> w37
          tunnel: w36 -> [w43 w48 w95 w113 w279 w428 w440 w442 w467 w488 w508 w527]
          tunnel: [w41 w47 w51 w106 w271 w434 w437 w460 w469 w485 w505 w526] -> w35
          event Timeout {
            n8 = event-data() -> ()  [unwired: 1 in, 1 out]
            n9 = call <vilib>:"Add State(s) to Queue__jki_lib_state_machine.vi"("State(s) in Front (\"\")"="" ("State(s) in Front (\"\")"), "State(s) in (\"\")"=w45) -> ("States Out"=w44:string)  [unwired: 13 in]
          }
          event Value Change {
            # "Exit Button Value Change (pressed) Event\n(this executes Macro: Exit to terminate the VI)"
            n10 = event-data() -> ()  [unwired: 1 in, 1 out]
            n11 = call <vilib>:"Add State(s) to Queue__jki_lib_state_machine.vi"("State(s) in Front (\"\")"="Get Main Info\nCheck Contents", "State(s) in (\"\")"=w50) -> ("States Out"=w49:string)  [unwired: 13 in]
          }
          event "Read Previous": Value Change {
            n12 = event-data() -> ()  [unwired: 1 in, 6 out]
            n13 = Unbundle By Name(w51) -> ("Filepath In.General Setup Paths.File Save Previous Run Path"=w92:path)
            n14 = call <vilib>:"Add State(s) to Queue__jki_lib_state_machine.vi"("State(s) in Front (\"\")"="Get Main Info\nGet Dish Info\nGet Washer Info", "State(s) in (\"\")"=w57) -> ("States Out"=w56:string)  [unwired: 13 in]
            n15 = call "Save File DOE Save Previous Input Data.vi"("State"=enum16{"Write", "Read"}."Read", "error in (no error)"=w95, "Appliance Previous Run Path"=w92) -> ("error out"=w94:errorcluster, "Appliance Details Ouput"=w91:T22)  [unwired: 7 in]
            n16 = Unbundle By Name(w91) -> ("Appliance Common.TR Number:"=w90:string, "Appliance Common.Lab ID:"=w89:string, "Appliance Common.Model Number:"=w88:string, "Appliance Common.Serial Number:"=w87:string, "Appliance Common.Station ID:"=w86:string, "Appliance Common.Engineer:"=w85:string, "Appliance Common.Technician:"=w84:string, "Appliance Common.Water Pressure (PSI):"=w83:string, "Appliance Common.Ambient RH:"=w82:string, "Appliance Common.Voltage:"=w81:string, "Appliance Common.Frequency:"=w80:string, "Appliance Common.Build:"=w79:string, "Appliance Common.Comments:"=w78:string, "Dishwasher Info.Manufacturer-Dish:"=w77:string, "Dishwasher Info.Unit Control-Dish:"=w76:string, "Appliance Common.Test Type:"=w75:string, "Dishwasher Info.Cycle Mode-Dish:"=w74:string, "Dishwasher Info.Inlet Temperature-Dish:"=w73:string, "Dishwasher Info.Detergent-Dish:"=w72:string, "Dishwasher Info.Auto Cup Weight (gm):"=w71:dbl, "Dishwasher Info.Open Cup Weight (gm):"=w70:dbl, "Washer Info.Model Family:"=w69:string, "Washer Info.Program Name:"=w68:string, "Washer Info.Cycle Selection:"=w67:string, "Washer Info.Wash Temperature:"=w66:string, "Washer Info.Rinse Temperature:"=w65:string, "Washer Info.Load Size:"=w64:string, "Washer Info.Hot Water Temperature (Fahrenheit):"=w63:string, "Washer Info.Cold Water Temperature (Fahrenheit):"=w62:string, "Washer Info.Capacity (cu.ft):"=w61:dbl, "Washer Info.Initial Cloth Weight:"=w60:dbl, "Washer Info.Cloth Lot:"=w59:i32, "Appliance Common.Load Run #:"=w58:i32, "Water Heater.Heating Mode:"=w53:string, "Appliance Common.Ambient Temperature (F):"=w52:string)
            n17 = local write "Manufacturer-Dish:"(w77) -> ()
            n18 = local write "Unit Control-Dish:"(w76) -> ()
            n19 = local write "Cycle Mode-Dish:"(w74) -> ()
            n20 = local write "Detergent-Dish:"(w72) -> ()
            n21 = local write "Inlet Temperature-Dish:"(w73) -> ()
            n22 = local write "Build:"(w79) -> ()
            n23 = local write "Comments:"(w78) -> ()
            n24 = local write "Auto Cup Weight (gm):"(w71) -> ()
            n25 = local write "Open Cup Weight (gm):"(w70) -> ()
            n26 = local write "Model Family"(w69) -> ()
            n27 = local write "Program Name"(w68) -> ()
            n28 = local write "Cycle Selection"(w67) -> ()
            n29 = local write "Wash Temperature"(w66) -> ()
            n30 = local write "Rinse Temperature"(w65) -> ()
            n31 = local write "Load Size"(w64) -> ()
            n32 = local write "Hot Water Temperature (Fahrenheit)"(w63) -> ()
            n33 = local write "Cold Water Temperature (Fahrenheit)"(w62) -> ()
            n34 = local write "Ambient RH:"(w82) -> ()
            n35 = local write "Supply Voltage:"(w81) -> ()
            n36 = local write "Frequency:"(w80) -> ()
            n37 = local write "Water Pressure (PSI):"(w83) -> ()
            n38 = local write "TR Number:"(w90) -> ()
            n39 = local write "Lab ID:"(w89) -> ()
            n40 = local write "Model:"(w88) -> ()
            n41 = local write "Serial Number:"(w87) -> ()
            n42 = local write "Station ID:"(w86) -> ()
            n43 = local write "Engineer:"(w85) -> ()
            n44 = local write "Technician:"(w84) -> ()
            n45 = local write "Test Type:"(w75) -> ()
            n46 = local write "Load Run #:"(w58) -> ()
            n47 = local write "Capacity (cu.ft)"(w61) -> ()
            n48 = local write "Initial Cloth Weight:"(w60) -> ()
            n49 = local write "Cloth Lot:"(w59) -> ()
            n50 = Unbundle By Name(w51) -> ("Filepath In"=w54:T10)
            n51 = local write "Ambient Temperature (F):"(w52) -> ()
            n52 = local write "Heating Mode"(w53) -> ()
            n53 = local write "Filepath In"(w54) -> ()
          }
          event "Remove Button 1", "Remove Button 2", "Remove Button 3", "Remove Button 4", "Remove Button 5", "Remove Button 6", "Remove Button 7", "Remove Button 8", "Remove Button 9", "Remove Button 10", "Remove Button 11", "Remove Button 12", "Remove Button 13", "Remove Button 14", "Remove Button 15", "Remove Button 16", "Remove Button 17", "Remove Button 18", "Remove Button 19", "Remove Button 20", "Remove Button 21", "Remove Button 22", "Remove Button 23", "Remove Button 24", "Remove Button 25", "Remove Button 26", "Remove Button 27", "Remove Button 28", "Remove Button 29", "Remove Button 30": Value Change {
            # "Populate the control\nwith the new values"
            n54 = event-data() -> ()  [unwired: 1 in, 6 out]
            n55 = Build Array("Remove Button 1", "Remove Button 2", "Remove Button 3", "Remove Button 4", "Remove Button 5", "Remove Button 6", "Remove Button 7", "Remove Button 8", "Remove Button 9", "Remove Button 10", "Remove Button 11", "Remove Button 12", "Remove Button 13", "Remove Button 14", "Remove Button 15", "Remove Button 16", "Remove Button 17", "Remove Button 18", "Remove Button 19", "Remove Button 20", "Remove Button 21", "Remove Button 22", "Remove Button 23", "Remove Button 24", "Remove Button 25", "Remove Button 26", "Remove Button 27", "Remove Button 28", "Remove Button 29", "Remove Button 30") -> (w117:bool[])
            n56 = for {
              tunnel: w117 -> [w170] mode=indexing
              shift-right: [w168] -> w112
              shift-left: w113 -> [w168]
              tunnel: [w167] -> w109
              tunnel: [w166] -> w111
              i -> [w169]
              stop <- w170 stop-if-true
              n57 = Increment(x=w169) -> (x+1=w167:i32)
              n58 = case shown="27" w167 {
                tunnel: [w171 w174 w177 w180 w183 w186 w190 w192 w195 w198 w201 w204 w207 w210 w213 w216 w219 w222 w225 w228 w232 w234 w237 w240 w243 w246 w250 w252 w255 w258] -> w166
                frame 1, Default {
                  # "Station ID Remove"
                  n59 = property on="Station ID:" class="CmbBox"() -> ("Label.Text"=w172:string)  [unwired: 2 in, 2 out]
                  n60 = local read "Station ID:"() -> (w173:string)
                  n61 = Build Array(w172, w173) -> (w171:string[])
                }
                frame 2 {
                  # "Technician Remove"
                  n62 = property on="Technician:" class="CmbBox"() -> ("Label.Text"=w175:string)  [unwired: 2 in, 2 out]
                  n63 = local read "Technician:"() -> (w176:string)
                  n64 = Build Array(w175, w176) -> (w174:string[])
                }
                frame 3 {
                  # "Water Pressure PSI Remove"
                  n65 = local read "Water Pressure (PSI):"() -> (w178:string)
                  n66 = property on="Water Pressure (PSI):" class="CmbBox"() -> ("Label.Text"=w179:string)  [unwired: 2 in, 2 out]
                  n67 = Build Array(w179, w178) -> (w177:string[])
                }
                frame 4 {
                  # "Ambient RH Remove"
                  n68 = property on="Ambient RH:" class="CmbBox"() -> ("Label.Text"=w182:string)  [unwired: 2 in, 2 out]
                  n69 = local read "Ambient RH:"() -> (w181:string)
                  n70 = Build Array(w182, w181) -> (w180:string[])
                }
                frame 5 {
                  # "Supply Voltage"
                  n71 = property on="Supply Voltage:" class="CmbBox"() -> ("Label.Text"=w184:string)  [unwired: 2 in, 2 out]
                  n72 = local read "Supply Voltage:"() -> (w185:string)
                  n73 = Build Array(w184, w185) -> (w183:string[])
                }
                frame 6 {
                  # "Frequency"
                  n74 = property on="Frequency:" class="CmbBox"() -> ("Label.Text"=w187:string)  [unwired: 2 in, 2 out]
                  n75 = local read "Frequency:"() -> (w188:string)
                  n76 = Build Array(w187, w188) -> (w186:string[])
                }
                frame 7 {
                  # "Build"
                  n77 = property on="Build:" class="CmbBox"() -> ("Label.Text"=w189:string)  [unwired: 2 in, 2 out]
                  n78 = local read "Build:"() -> (w191:string)
                  n79 = Build Array(w189, w191) -> (w190:string[])
                }
                frame 8 {
                  # "Hot Water Temperature (Washer)"
                  n80 = local read "Hot Water Temperature (Fahrenheit)"() -> (w194:string)
                  n81 = property on="Hot Water Temperature (Fahrenheit)" class="CmbBox"() -> ("Label.Text"=w193:string)  [unwired: 2 in, 2 out]
                  n82 = Build Array(w193, w194) -> (w192:string[])
                }
                frame 9 {
                  # "Cold Water Temperature (Washer)"
                  n83 = property on="Cold Water Temperature (Fahrenheit)" class="CmbBox"() -> ("Label.Text"=w196:string)  [unwired: 2 in, 2 out]
                  n84 = local read "Cold Water Temperature (Fahrenheit)"() -> (w197:string)
                  n85 = Build Array(w196, w197) -> (w195:string[])
                }
                frame 10 {
                  # "Manufacturer (Dish)"
                  n86 = local read "Manufacturer-Dish:"() -> (w200:string)
                  n87 = property on="Manufacturer-Dish:" class="CmbBox"() -> ("Label.Text"=w199:string)  [unwired: 2 in, 2 out]
                  n88 = Build Array(w199, w200) -> (w198:string[])
                }
                frame 11 {
                  # "Unit Control (Dish)"
                  n89 = local read "Unit Control-Dish:"() -> (w202:string)
                  n90 = property on="Unit Control-Dish:" class="CmbBox"() -> ("Label.Text"=w203:string)  [unwired: 2 in, 2 out]
                  n91 = Build Array(w203, w202) -> (w201:string[])
                }
                frame 12 {
                  # "Test Type (Dish)"
                  n92 = property on="Test Type:" class="CmbBox"() -> ("Label.Text"=w205:string)  [unwired: 2 in, 2 out]
                  n93 = local read "Test Type:"() -> (w206:string)
                  n94 = Build Array(w205, w206) -> (w204:string[])
                }
                frame 13 {
                  # "Cycle Mode (Dish)"
                  n95 = local read "Cycle Mode-Dish:"() -> (w209:string)
                  n96 = property on="Cycle Mode-Dish:" class="CmbBox"() -> ("Label.Text"=w208:string)  [unwired: 2 in, 2 out]
                  n97 = Build Array(w208, w209) -> (w207:string[])
                }
                frame 14 {
                  # "Inlet Temperature (Dish)"
                  n98 = local read "Inlet Temperature-Dish:"() -> (w212:string)
                  n99 = property on="Inlet Temperature-Dish:" class="CmbBox"() -> ("Label.Text"=w211:string)  [unwired: 2 in, 2 out]
                  n100 = Build Array(w211, w212) -> (w210:string[])
                }
                frame 15 {
                  # "Detergent (Dish)"
                  n101 = local read "Detergent-Dish:"() -> (w215:string)
                  n102 = property on="Detergent-Dish:" class="CmbBox"() -> ("Label.Text"=w214:string)  [unwired: 2 in, 2 out]
                  n103 = Build Array(w214, w215) -> (w213:string[])
                }
                frame 16 {
                  # "TR Number"
                  n104 = property on="TR Number:" class="CmbBox"() -> ("Label.Text"=w217:string)  [unwired: 2 in, 2 out]
                  n105 = local read "TR Number:"() -> (w218:string)
                  n106 = Build Array(w217, w218) -> (w216:string[])
                }
                frame 17 {
                  # "Lab ID Number"
                  n107 = property on="Lab ID:" class="CmbBox"() -> ("Label.Text"=w220:string)  [unwired: 2 in, 2 out]
                  n108 = local read "Lab ID:"() -> (w221:string)
                  n109 = Build Array(w220, w221) -> (w219:string[])
                }
                frame 18 {
                  n110 = property on="Wash Temperature" class="CmbBox"() -> ("Label.Text"=w223:string)  [unwired: 2 in, 2 out]
                  n111 = local read "Wash Temperature"() -> (w224:string)
                  n112 = Build Array(w223, w224) -> (w222:string[])
                }
                frame 19 {
                  n113 = property on="Rinse Temperature" class="CmbBox"() -> ("Label.Text"=w226:string)  [unwired: 2 in, 2 out]
                  n114 = local read "Rinse Temperature"() -> (w227:string)
                  n115 = Build Array(w226, w227) -> (w225:string[])
                }
                frame 20 {
                  n116 = property on="Load Size" class="CmbBox"() -> ("Label.Text"=w229:string)  [unwired: 2 in, 2 out]
                  n117 = local read "Load Size"() -> (w230:string)
                  n118 = Build Array(w229, w230) -> (w228:string[])
                }
                frame 21 {
                  n119 = property on="Cycle Selection" class="CmbBox"() -> ("Label.Text"=w231:string)  [unwired: 2 in, 2 out]
                  n120 = local read "Cycle Selection"() -> (w233:string)
                  n121 = Build Array(w231, w233) -> (w232:string[])
                }
                frame 22 {
                  n122 = property on="Heating Mode" class="CmbBox (strict)"() -> ("Label.Text"=w235:string)  [unwired: 2 in, 2 out]
                  n123 = local read "Heating Mode"() -> (w236:T4)
                  n124 = Build Array(w235, w236) -> (w234:T4[])
                }
                frame 23 {
                  n125 = local read "Ambient Temperature (F):"() -> (w238:string)
                  n126 = property on="Ambient Temperature (F):" class="CmbBox"() -> ("Label.Text"=w239:string)  [unwired: 2 in, 2 out]
                  n127 = Build Array(w239, w238) -> (w237:string[])
                }
                frame 24 {
                  n128 = local read "Dryer Type:"() -> (w241:string)
                  n129 = property on="Dryer Type:" class="CmbBox"() -> ("Label.Text"=w242:string)  [unwired: 2 in, 2 out]
                  n130 = Build Array(w242, w241) -> (w240:string[])
                }
                frame 25 {
                  n131 = local read "Exhaust:"() -> (w244:string)
                  n132 = property on="Exhaust:" class="CmbBox"() -> ("Label.Text"=w245:string)  [unwired: 2 in, 2 out]
                  n133 = Build Array(w245, w244) -> (w243:string[])
                }
                frame 26 {
                  n134 = local read "Drying Cycle:"() -> (w247:string)
                  n135 = property on="Drying Cycle:" class="CmbBox"() -> ("Label.Text"=w248:string)  [unwired: 2 in, 2 out]
                  n136 = Build Array(w248, w247) -> (w246:string[])
                }
                frame 27 {
                  n137 = local read "Heat Setting:"() -> (w249:string)
                  n138 = property on="Heat Setting:" class="CmbBox"() -> ("Label.Text"=w251:string)  [unwired: 2 in, 2 out]
                  n139 = Build Array(w251, w249) -> (w250:string[])
                }
                frame 28 {
                  n140 = local read "Dryness Setting:"() -> (w253:string)
                  n141 = property on="Dryness Setting:" class="CmbBox"() -> ("Label.Text"=w254:string)  [unwired: 2 in, 2 out]
                  n142 = Build Array(w254, w253) -> (w252:string[])
                }
                frame 29 {
                  n143 = local read "Nominal Load Weight (lbs):"() -> (w256:string)
                  n144 = property on="Nominal Load Weight (lbs):" class="CmbBox"() -> ("Label.Text"=w257:string)  [unwired: 2 in, 2 out]
                  n145 = Build Array(w257, w256) -> (w255:string[])
                }
                frame 30 {
                  n146 = local read "Load Type:"() -> (w259:string)
                  n147 = property on="Load Type:" class="CmbBox"() -> ("Label.Text"=w260:string)  [unwired: 2 in, 2 out]
                  n148 = Build Array(w260, w259) -> (w258:string[])
                }
              }
            }
            n149 = Unbundle By Name(w106) -> ("Filepath In.General Setup Paths.File Save Configuration Data Path"=w105:path)
            n150 = call "Save File DOE Configuration.vi"("Add/Remove Enum"=T27."Remove", "Latest String Search"=w111, "error in (no error)"=w112, "File Save Configuration Data Path"=w105) -> ("error out"=w120:errorcluster, "Updated List"=w108:string[])  [unwired: 5 in, 1 out]
            n151 = case shown="22" w109 {
              tunnel: w108 -> [w137 w138 w139 w140 w141 w142 w143 w144 w145 w146 w147 w148 w149 w150 w151 w152 w153 w154 w155 w156 w157 _ w158 w159 w160 w161 w162 w163 w164 w165]
              frame 1, Default {
                n152 = property on="Station ID:" class="CmbBox"("Strings[]"=w137) -> ()  [unwired: 2 in, 2 out]
              }
              frame 2 {
                n153 = property on="Technician:" class="CmbBox"("Strings[]"=w138) -> ()  [unwired: 2 in, 2 out]
              }
              frame 3 {
                n154 = property on="Water Pressure (PSI):" class="CmbBox"("Strings[]"=w139) -> ()  [unwired: 2 in, 2 out]
              }
              frame 4 {
                n155 = property on="Ambient RH:" class="CmbBox"("Strings[]"=w140) -> ()  [unwired: 2 in, 2 out]
              }
              frame 5 {
                n156 = property on="Supply Voltage:" class="CmbBox"("Strings[]"=w141) -> ()  [unwired: 2 in, 2 out]
              }
              frame 6 {
                n157 = property on="Frequency:" class="CmbBox"("Strings[]"=w142) -> ()  [unwired: 2 in, 2 out]
              }
              frame 7 {
                n158 = property on="Build:" class="CmbBox"("Strings[]"=w143) -> ()  [unwired: 2 in, 2 out]
              }
              frame 8 {
                n159 = property on="Hot Water Temperature (Fahrenheit)" class="CmbBox"("Strings[]"=w144) -> ()  [unwired: 2 in, 2 out]
              }
              frame 9 {
                n160 = property on="Cold Water Temperature (Fahrenheit)" class="CmbBox"("Strings[]"=w145) -> ()  [unwired: 2 in, 2 out]
              }
              frame 10 {
                n161 = property on="Manufacturer-Dish:" class="CmbBox"("Strings[]"=w146) -> ()  [unwired: 2 in, 2 out]
              }
              frame 11 {
                n162 = property on="Unit Control-Dish:" class="CmbBox"("Strings[]"=w147) -> ()  [unwired: 2 in, 2 out]
              }
              frame 12 {
                n163 = property on="Test Type:" class="CmbBox"("Strings[]"=w148) -> ()  [unwired: 2 in, 2 out]
              }
              frame 13 {
                n164 = property on="Cycle Mode-Dish:" class="CmbBox"("Strings[]"=w149) -> ()  [unwired: 2 in, 2 out]
              }
              frame 14 {
                n165 = property on="Inlet Temperature-Dish:" class="CmbBox"("Strings[]"=w150) -> ()  [unwired: 2 in, 2 out]
              }
              frame 15 {
                n166 = property on="Detergent-Dish:" class="CmbBox"("Strings[]"=w151) -> ()  [unwired: 2 in, 2 out]
              }
              frame 16 {
                n167 = property on="TR Number:" class="CmbBox"("Strings[]"=w152) -> ()  [unwired: 2 in, 2 out]
              }
              frame 17 {
                n168 = property on="Lab ID:" class="CmbBox"("Strings[]"=w153) -> ()  [unwired: 2 in, 2 out]
              }
              frame 18 {
                n169 = property on="Wash Temperature" class="CmbBox"("Strings[]"=w154) -> ()  [unwired: 2 in, 2 out]
              }
              frame 19 {
                n170 = property on="Rinse Temperature" class="CmbBox"("Strings[]"=w155) -> ()  [unwired: 2 in, 2 out]
              }
              frame 20 {
                n171 = property on="Load Size" class="CmbBox"("Strings[]"=w156) -> ()  [unwired: 2 in, 2 out]
              }
              frame 21 {
                n172 = property on="Cycle Selection" class="CmbBox"("Strings[]"=w157) -> ()  [unwired: 2 in, 2 out]
              }
              frame 22 {
              }
              frame 23 {
                n173 = property on="Ambient Temperature (F):" class="CmbBox"("Strings[]"=w158) -> ()  [unwired: 2 in, 2 out]
              }
              frame 24 {
                n174 = property on="Dryer Type:" class="CmbBox"("Strings[]"=w159) -> ()  [unwired: 2 in, 2 out]
              }
              frame 25 {
                n175 = property on="Exhaust:" class="CmbBox"("Strings[]"=w160) -> ()  [unwired: 2 in, 2 out]
              }
              frame 26 {
                n176 = property on="Drying Cycle:" class="CmbBox"("Strings[]"=w161) -> ()  [unwired: 2 in, 2 out]
              }
              frame 27 {
                n177 = property on="Heat Setting:" class="CmbBox"("Strings[]"=w162) -> ()  [unwired: 2 in, 2 out]
              }
              frame 28 {
                n178 = property on="Dryness Setting:" class="CmbBox"("Strings[]"=w163) -> ()  [unwired: 2 in, 2 out]
              }
              frame 29 {
                n179 = property on="Nominal Load Weight (lbs):" class="CmbBox"("Strings[]"=w164) -> ()  [unwired: 2 in, 2 out]
              }
              frame 30 {
                n180 = property on="Load Type:" class="CmbBox"("Strings[]"=w165) -> ()  [unwired: 2 in, 2 out]
              }
            }
          }
          event "Add Button 1", "Add Button 2", "Add Button 3", "Add Button 4", "Add Button 5", "Add Button 6", "Add Button 7", "Add Button 8", "Add Button 9", "Add Button 10", "Add Button 11", "Add Button 12", "Add Button 13", "Add Button 14", "Add Button 15", "Add Button 16", "Add Button 17", "Add Button 18", "Add Button 19", "Add Button 20", "Add Button 21", "Add Button 22", "Add Button 23", "Add Button 24", "Add Button 25", "Add Button 26", "Add Button 27", "Add Button 28", "Add Button 29", "Add Button 30": Value Change {
            n181 = event-data() -> ()  [unwired: 1 in, 6 out]
            n182 = Build Array("Add Button 1", "Add Button 2", "Add Button 3", "Add Button 4", "Add Button 5", "Add Button 6", "Add Button 7", "Add Button 8", "Add Button 9", "Add Button 10", "Add Button 11", "Add Button 12", "Add Button 13", "Add Button 14", "Add Button 15", "Add Button 16", "Add Button 17", "Add Button 18", "Add Button 19", "Add Button 20", "Add Button 21", "Add Button 22", "Add Button 23", "Add Button 24", "Add Button 25", "Add Button 26", "Add Button 27", "Add Button 28", "Add Button 29", "Add Button 30") -> (w280:bool[])
            n183 = for {
              tunnel: w280 -> [w335] mode=indexing
              shift-right: [w333] -> w278
              shift-left: w279 -> [w333]
              tunnel: [w331] -> w273
              tunnel: [w332] -> w276
              i -> [w334]
              stop <- w335 stop-if-true
              n184 = Increment(x=w334) -> (x+1=w331:i32)
              n185 = case shown="23" w331 {
                tunnel: [w336 w339 w342 w345 w348 w351 w355 w357 w360 w363 w366 w369 w372 w375 w378 w381 w384 w387 w390 w393 w397 w399 w402 w405 w408 w411 w416 w419 w421 w424] -> w332
                frame 1, Default {
                  # "Station ID Remove"
                  n186 = property on="Station ID:" class="CmbBox"() -> ("Label.Text"=w337:string)  [unwired: 2 in, 2 out]
                  n187 = local read "Station ID:"() -> (w338:string)
                  n188 = Build Array(w337, w338) -> (w336:string[])
                }
                frame 2 {
                  # "Technician Remove"
                  n189 = property on="Technician:" class="CmbBox"() -> ("Label.Text"=w340:string)  [unwired: 2 in, 2 out]
                  n190 = local read "Technician:"() -> (w341:string)
                  n191 = Build Array(w340, w341) -> (w339:string[])
                }
                frame 3 {
                  # "Water Pressure PSI Remove"
                  n192 = local read "Water Pressure (PSI):"() -> (w343:string)
                  n193 = property on="Water Pressure (PSI):" class="CmbBox"() -> ("Label.Text"=w344:string)  [unwired: 2 in, 2 out]
                  n194 = Build Array(w344, w343) -> (w342:string[])
                }
                frame 4 {
                  # "Ambient RH Remove"
                  n195 = property on="Ambient RH:" class="CmbBox"() -> ("Label.Text"=w347:string)  [unwired: 2 in, 2 out]
                  n196 = local read "Ambient RH:"() -> (w346:string)
                  n197 = Build Array(w347, w346) -> (w345:string[])
                }
                frame 5 {
                  # "Supply Voltage"
                  n198 = property on="Supply Voltage:" class="CmbBox"() -> ("Label.Text"=w349:string)  [unwired: 2 in, 2 out]
                  n199 = local read "Supply Voltage:"() -> (w350:string)
                  n200 = Build Array(w349, w350) -> (w348:string[])
                }
                frame 6 {
                  # "Frequency"
                  n201 = property on="Frequency:" class="CmbBox"() -> ("Label.Text"=w352:string)  [unwired: 2 in, 2 out]
                  n202 = local read "Frequency:"() -> (w353:string)
                  n203 = Build Array(w352, w353) -> (w351:string[])
                }
                frame 7 {
                  # "Build"
                  n204 = property on="Build:" class="CmbBox"() -> ("Label.Text"=w354:string)  [unwired: 2 in, 2 out]
                  n205 = local read "Build:"() -> (w356:string)
                  n206 = Build Array(w354, w356) -> (w355:string[])
                }
                frame 8 {
                  # "Hot Water Temperature (Washer)"
                  n207 = local read "Hot Water Temperature (Fahrenheit)"() -> (w359:string)
                  n208 = property on="Hot Water Temperature (Fahrenheit)" class="CmbBox"() -> ("Label.Text"=w358:string)  [unwired: 2 in, 2 out]
                  n209 = Build Array(w358, w359) -> (w357:string[])
                }
                frame 9 {
                  # "Cold Water Temperature (Washer)"
                  n210 = property on="Cold Water Temperature (Fahrenheit)" class="CmbBox"() -> ("Label.Text"=w361:string)  [unwired: 2 in, 2 out]
                  n211 = local read "Cold Water Temperature (Fahrenheit)"() -> (w362:string)
                  n212 = Build Array(w361, w362) -> (w360:string[])
                }
                frame 10 {
                  # "Manufacturer (Dish)"
                  n213 = local read "Manufacturer-Dish:"() -> (w365:string)
                  n214 = property on="Manufacturer-Dish:" class="CmbBox"() -> ("Label.Text"=w364:string)  [unwired: 2 in, 2 out]
                  n215 = Build Array(w364, w365) -> (w363:string[])
                }
                frame 11 {
                  # "Unit Control (Dish)"
                  n216 = local read "Unit Control-Dish:"() -> (w367:string)
                  n217 = property on="Unit Control-Dish:" class="CmbBox"() -> ("Label.Text"=w368:string)  [unwired: 2 in, 2 out]
                  n218 = Build Array(w368, w367) -> (w366:string[])
                }
                frame 12 {
                  # "Test Type"
                  n219 = property on="Test Type:" class="CmbBox"() -> ("Label.Text"=w370:string)  [unwired: 2 in, 2 out]
                  n220 = local read "Test Type:"() -> (w371:string)
                  n221 = Build Array(w370, w371) -> (w369:string[])
                }
                frame 13 {
                  # "Cycle Mode (Dish)"
                  n222 = local read "Cycle Mode-Dish:"() -> (w374:string)
                  n223 = property on="Cycle Mode-Dish:" class="CmbBox"() -> ("Label.Text"=w373:string)  [unwired: 2 in, 2 out]
                  n224 = Build Array(w373, w374) -> (w372:string[])
                }
                frame 14 {
                  # "Inlet Temperature (Dish)"
                  n225 = local read "Inlet Temperature-Dish:"() -> (w377:string)
                  n226 = property on="Inlet Temperature-Dish:" class="CmbBox"() -> ("Label.Text"=w376:string)  [unwired: 2 in, 2 out]
                  n227 = Build Array(w376, w377) -> (w375:string[])
                }
                frame 15 {
                  # "Detergent (Dish)"
                  n228 = local read "Detergent-Dish:"() -> (w380:string)
                  n229 = property on="Detergent-Dish:" class="CmbBox"() -> ("Label.Text"=w379:string)  [unwired: 2 in, 2 out]
                  n230 = Build Array(w379, w380) -> (w378:string[])
                }
                frame 16 {
                  # "TR Number"
                  n231 = property on="TR Number:" class="CmbBox"() -> ("Label.Text"=w382:string)  [unwired: 2 in, 2 out]
                  n232 = local read "TR Number:"() -> (w383:string)
                  n233 = Build Array(w382, w383) -> (w381:string[])
                }
                frame 17 {
                  # "Lab ID Number"
                  n234 = property on="Lab ID:" class="CmbBox"() -> ("Label.Text"=w385:string)  [unwired: 2 in, 2 out]
                  n235 = local read "Lab ID:"() -> (w386:string)
                  n236 = Build Array(w385, w386) -> (w384:string[])
                }
                frame 18 {
                  n237 = property on="Wash Temperature" class="CmbBox"() -> ("Label.Text"=w388:string)  [unwired: 2 in, 2 out]
                  n238 = local read "Wash Temperature"() -> (w389:string)
                  n239 = Build Array(w388, w389) -> (w387:string[])
                }
                frame 19 {
                  n240 = property on="Rinse Temperature" class="CmbBox"() -> ("Label.Text"=w391:string)  [unwired: 2 in, 2 out]
                  n241 = local read "Rinse Temperature"() -> (w392:string)
                  n242 = Build Array(w391, w392) -> (w390:string[])
                }
                frame 20 {
                  n243 = property on="Load Size" class="CmbBox"() -> ("Label.Text"=w394:string)  [unwired: 2 in, 2 out]
                  n244 = local read "Load Size"() -> (w395:string)
                  n245 = Build Array(w394, w395) -> (w393:string[])
                }
                frame 21 {
                  n246 = property on="Cycle Selection" class="CmbBox"() -> ("Label.Text"=w396:string)  [unwired: 2 in, 2 out]
                  n247 = local read "Cycle Selection"() -> (w398:string)
                  n248 = Build Array(w396, w398) -> (w397:string[])
                }
                frame 22 {
                  n249 = property on="Heating Mode" class="CmbBox (strict)"() -> ("Label.Text"=w400:string)  [unwired: 2 in, 2 out]
                  n250 = local read "Heating Mode"() -> (w401:T4)
                  n251 = Build Array(w400, w401) -> (w399:T4[])
                }
                frame 23 {
                  n252 = local read "Ambient Temperature (F):"() -> (w403:string)
                  n253 = property on="Ambient Temperature (F):" class="CmbBox"() -> ("Label.Text"=w404:string)  [unwired: 2 in, 2 out]
                  n254 = Build Array(w404, w403) -> (w402:string[])
                }
                frame 24 {
                  n255 = local read "Dryer Type:"() -> (w406:string)
                  n256 = property on="Dryer Type:" class="CmbBox"() -> ("Label.Text"=w407:string)  [unwired: 2 in, 2 out]
                  n257 = Build Array(w407, w406) -> (w405:string[])
                }
                frame 25 {
                  n258 = local read "Exhaust:"() -> (w409:string)
                  n259 = property on="Exhaust:" class="CmbBox"() -> ("Label.Text"=w410:string)  [unwired: 2 in, 2 out]
                  n260 = Build Array(w410, w409) -> (w408:string[])
                }
                frame 26 {
                  n261 = local read "Drying Cycle:"() -> (w412:string)
                  n262 = property on="Drying Cycle:" class="CmbBox"() -> ("Label.Text"=w413:string)  [unwired: 2 in, 2 out]
                  n263 = Build Array(w413, w412) -> (w411:string[])
                }
                frame 27 {
                  n264 = local read "Heat Setting:"() -> (w414:string)
                  n265 = property on="Heat Setting:" class="CmbBox"() -> ("Label.Text"=w415:string)  [unwired: 2 in, 2 out]
                  n266 = Build Array(w415, w414) -> (w416:string[])
                }
                frame 28 {
                  n267 = local read "Dryness Setting:"() -> (w417:string)
                  n268 = property on="Dryness Setting:" class="CmbBox"() -> ("Label.Text"=w418:string)  [unwired: 2 in, 2 out]
                  n269 = Build Array(w418, w417) -> (w419:string[])
                }
                frame 29 {
                  n270 = local read "Nominal Load Weight (lbs):"() -> (w420:string)
                  n271 = property on="Nominal Load Weight (lbs):" class="CmbBox"() -> ("Label.Text"=w422:string)  [unwired: 2 in, 2 out]
                  n272 = Build Array(w422, w420) -> (w421:string[])
                }
                frame 30 {
                  n273 = local read "Load Type:"() -> (w423:string)
                  n274 = property on="Load Type:" class="CmbBox"() -> ("Label.Text"=w425:string)  [unwired: 2 in, 2 out]
                  n275 = Build Array(w425, w423) -> (w424:string[])
                }
              }
            }
            n276 = Unbundle By Name(w271) -> ("Filepath In.General Setup Paths.File Save Configuration Data Path"=w270:path)
            n277 = call "Save File DOE Configuration.vi"("Add/Remove Enum"=T27."Add", "Latest String Search"=w276, "error in (no error)"=w278, "File Save Configuration Data Path"=w270, "Button Number"=w273) -> ("error out"=w277:errorcluster, "Updated List"=w274:string[])  [unwired: 4 in, 1 out]
            n278 = case shown="22" w273 {
              tunnel: w274 -> [w302 w303 w304 w305 w306 w307 w308 w309 w310 w311 w312 w313 w314 w315 w316 w317 w318 w319 w320 w321 w322 _ w323 w324 w325 w326 w327 w328 w329 w330]
              frame 1, Default {
                n279 = property on="Station ID:" class="CmbBox"("Strings[]"=w302) -> ()  [unwired: 2 in, 2 out]
              }
              frame 2 {
                n280 = property on="Technician:" class="CmbBox"("Strings[]"=w303) -> ()  [unwired: 2 in, 2 out]
              }
              frame 3 {
                n281 = property on="Water Pressure (PSI):" class="CmbBox"("Strings[]"=w304) -> ()  [unwired: 2 in, 2 out]
              }
              frame 4 {
                n282 = property on="Ambient RH:" class="CmbBox"("Strings[]"=w305) -> ()  [unwired: 2 in, 2 out]
              }
              frame 5 {
                n283 = property on="Supply Voltage:" class="CmbBox"("Strings[]"=w306) -> ()  [unwired: 2 in, 2 out]
              }
              frame 6 {
                n284 = property on="Frequency:" class="CmbBox"("Strings[]"=w307) -> ()  [unwired: 2 in, 2 out]
              }
              frame 7 {
                n285 = property on="Build:" class="CmbBox"("Strings[]"=w308) -> ()  [unwired: 2 in, 2 out]
              }
              frame 8 {
                n286 = property on="Hot Water Temperature (Fahrenheit)" class="CmbBox"("Strings[]"=w309) -> ()  [unwired: 2 in, 2 out]
              }
              frame 9 {
                n287 = property on="Cold Water Temperature (Fahrenheit)" class="CmbBox"("Strings[]"=w310) -> ()  [unwired: 2 in, 2 out]
              }
              frame 10 {
                n288 = property on="Manufacturer-Dish:" class="CmbBox"("Strings[]"=w311) -> ()  [unwired: 2 in, 2 out]
              }
              frame 11 {
                n289 = property on="Unit Control-Dish:" class="CmbBox"("Strings[]"=w312) -> ()  [unwired: 2 in, 2 out]
              }
              frame 12 {
                n290 = property on="Test Type:" class="CmbBox"("Strings[]"=w313) -> ()  [unwired: 2 in, 2 out]
              }
              frame 13 {
                n291 = property on="Cycle Mode-Dish:" class="CmbBox"("Strings[]"=w314) -> ()  [unwired: 2 in, 2 out]
              }
              frame 14 {
                n292 = property on="Inlet Temperature-Dish:" class="CmbBox"("Strings[]"=w315) -> ()  [unwired: 2 in, 2 out]
              }
              frame 15 {
                n293 = property on="Detergent-Dish:" class="CmbBox"("Strings[]"=w316) -> ()  [unwired: 2 in, 2 out]
              }
              frame 16 {
                n294 = property on="TR Number:" class="CmbBox"("Strings[]"=w317) -> ()  [unwired: 2 in, 2 out]
              }
              frame 17 {
                n295 = property on="Lab ID:" class="CmbBox"("Strings[]"=w318) -> ()  [unwired: 2 in, 2 out]
              }
              frame 18 {
                n296 = property on="Wash Temperature" class="CmbBox"("Strings[]"=w319) -> ()  [unwired: 2 in, 2 out]
              }
              frame 19 {
                n297 = property on="Rinse Temperature" class="CmbBox"("Strings[]"=w320) -> ()  [unwired: 2 in, 2 out]
              }
              frame 20 {
                n298 = property on="Load Size" class="CmbBox"("Strings[]"=w321) -> ()  [unwired: 2 in, 2 out]
              }
              frame 21 {
                n299 = property on="Cycle Selection" class="CmbBox"("Strings[]"=w322) -> ()  [unwired: 2 in, 2 out]
              }
              frame 22 {
              }
              frame 23 {
                n300 = property on="Ambient Temperature (F):" class="CmbBox"("Strings[]"=w323) -> ()  [unwired: 2 in, 2 out]
              }
              frame 24 {
                n301 = property on="Dryer Type:" class="CmbBox"("Strings[]"=w324) -> ()  [unwired: 2 in, 2 out]
              }
              frame 25 {
                n302 = property on="Exhaust:" class="CmbBox"("Strings[]"=w325) -> ()  [unwired: 2 in, 2 out]
              }
              frame 26 {
                n303 = property on="Drying Cycle:" class="CmbBox"("Strings[]"=w326) -> ()  [unwired: 2 in, 2 out]
              }
              frame 27 {
                n304 = property on="Heat Setting:" class="CmbBox"("Strings[]"=w327) -> ()  [unwired: 2 in, 2 out]
              }
              frame 28 {
                n305 = property on="Dryness Setting:" class="CmbBox"("Strings[]"=w328) -> ()  [unwired: 2 in, 2 out]
              }
              frame 29 {
                n306 = property on="Nominal Load Weight (lbs):" class="CmbBox"("Strings[]"=w329) -> ()  [unwired: 2 in, 2 out]
              }
              frame 30 {
                n307 = property on="Load Type:" class="CmbBox"("Strings[]"=w330) -> ()  [unwired: 2 in, 2 out]
              }
            }
          }
          event "Initialize Default": Value Change {
            # "Read the default config file"
            # "Write default values to the main Config File"
            # "Send it back to load configuration to \npopulate the controls"
            n308 = event-data() -> ()  [unwired: 1 in, 6 out]
            n309 = Unbundle By Name(w434) -> ("Filepath In.General Setup Paths.General Startup Config Path"=w429:path)
            n310 = call "Save File DOE Reinitialize Drop Downs to Default.vi"("Save Default"=enum16{"Standard", "Save To Default"}."Standard") -> ("Default Data"=w426:string[][])  [unwired: 9 in, 1 out]
            n311 = call-poly <vilib>:"Write To Spreadsheet File.vi"("delimiter (\\t)"="," ("delimiter (\\t)"), "2D data"=w426, "file path (dialog if empty)"=w429) -> ()  [unwired: 5 in, 1 out]
            n312 = call <vilib>:"Add State(s) to Queue__jki_lib_state_machine.vi"("State(s) in Front (\"\")"="Load Configuration" ("State(s) in Front (\"\")"), "State(s) in (\"\")"=w433) -> ("States Out"=w432:string)  [unwired: 13 in]
          }
          event "Save As Default": Value Change {
            # "Read the default config file"
            n313 = event-data() -> ()  [unwired: 1 in, 6 out]
            n314 = Unbundle By Name(w437) -> ("Filepath In.General Setup Paths.General Startup Config Path"=w436:path)
            n315 = call "Save File DOE Reinitialize Drop Downs to Default.vi"("Save Default"=enum16{"Standard", "Save To Default"}."Save To Default", "error in (no error)"=w440, "Standard Path"=w436) -> ("error out"=w439:errorcluster)  [unwired: 7 in, 1 out]
          }
          event "Get Data": Value Change {
            n316 = event-data() -> ()  [unwired: 1 in, 6 out]
            n317 = Unbundle By Name(w459) -> ("Washer Controls In.Initialize.Washer In.Appliance Details.Dryer.Dryer Initial IMC Data"=w457:T25, "Washer Controls In.Test Fixture Hardware.Weight Scale.Com Options.Setra Scale VISA"=w451:refnum<visa-resource-name>)
            n318 = call "Setra Main.vi"("VISA resource name"=w451, "Runtime Gather?"=TRUE, "Error In"=w442) -> ("Weight Output"=w446:dbl, "Error Out"=w441:errorcluster)  [unwired: 10 in, 1 out]
            n319 = property on="Measured Weight (lbf)" class="DigNum (strict)"("Value"=w446) -> ()  [unwired: 2 in, 2 out]
            n320 = Bundle By Name(cluster=w457, "Bone Dry Wt(lbs)"="Bone Dry Weight (lbf)", "RMC (Desired %)"="Relative Moisture (%)", "Tolerance(%)"="Tolerance (%)", "Measured IMC (lbs)"=w446) -> (w456:T25)
            n321 = call "Save File DPT RMC Calculations.vi"("Dryer IMC Data Input"=w456, "Error In"=w441) -> ("Dryer IMC Data Output"=w455:T25, "Error Out"=w445:errorcluster)  [unwired: 16 in]
            n322 = Unbundle By Name(w455) -> ("Minimum Weight (lbf)"=→"Minimum Weight (lbf)":dbl, "Average Weight (lbf)"=→"Average Weight (lbf)":dbl, "Maximum Weight (lbf)"=→"Maximum Weight (lbf)":dbl, "Actual Initial RMC (%)"=→"Measured Conent (%)":dbl, "Measured IMC In Range?"=w443:bool)
            n323 = Bundle By Name(cluster=w459, "Washer Controls In.Initialize.Washer In.Appliance Details.Dryer.Dryer Initial IMC Data"=w455) -> (w460:T31)
            n324 = case shown="True" w443 {
              tunnel: ["Out of Range" "In Range"] -> w444
              frame False {
              }
              frame True {
              }
            }
            n325 = local write "In Range?"(w444) -> ()
          }
          event "Bone Dry Weight (lbf)", "Relative Moisture (%)", "Tolerance (%)", "Measured Weight (lbf)": Value Change {
            n326 = event-data() -> ()  [unwired: 1 in, 6 out]
            n327 = local read "Bone Dry Weight (lbf)"() -> (w474:dbl)
            n328 = local read "Relative Moisture (%)"() -> (w475:dbl)
            n329 = local read "Tolerance (%)"() -> (w476:dbl)
            n330 = Unbundle By Name(w470) -> ("Washer Controls In.Initialize.Washer In.Appliance Details.Dryer.Dryer Initial IMC Data"=w473:T25)
            n331 = property on="Measured Weight (lbf)" class="DigNum (strict)"() -> ("Value"=w481:dbl)  [unwired: 2 in, 2 out]
            n332 = Bundle By Name(cluster=w473, "Bone Dry Wt(lbs)"=w474, "RMC (Desired %)"=w475, "Tolerance(%)"=w476, "Measured IMC (lbs)"=w481) -> (w472:T25)
            n333 = call "Save File DPT RMC Calculations.vi"("Dryer IMC Data Input"=w472, "Error In"=w467) -> ("Dryer IMC Data Output"=w471:T25, "Error Out"=w466:errorcluster)  [unwired: 16 in]
            n334 = Unbundle By Name(w471) -> ("Minimum Weight (lbf)"=w477:dbl, "Average Weight (lbf)"=w478:dbl, "Maximum Weight (lbf)"=w479:dbl, "Actual Initial RMC (%)"=w480:dbl, "Measured IMC In Range?"=w465:bool)
            n335 = Bundle By Name(cluster=w470, "Washer Controls In.Initialize.Washer In.Appliance Details.Dryer.Dryer Initial IMC Data"=w471) -> (w469:T31)
            n336 = case shown="True" w465 {
              tunnel: ["Out of Range" "In Range"] -> w464
              frame False {
              }
              frame True {
              }
            }
            "In Range?" <- w464
            n337 = local write "Minimum Weight (lbf)"(w477) -> ()
            n338 = local write "Average Weight (lbf)"(w478) -> ()
            n339 = local write "Maximum Weight (lbf)"(w479) -> ()
            n340 = local write "Measured Conent (%)"(w480) -> ()
          }
          event "Get Weigth": Value Change {
            n341 = event-data() -> ()  [unwired: 1 in, 6 out]
            n342 = Unbundle By Name(w485) -> ("Washer Controls In.Test Fixture Hardware.Weight Scale.Select Scale"=w484:string)
            n343 = case shown="\"IND560 SERIAL\"" w484 {
              tunnel: w485 -> [w493 w503]
              tunnel: [w495 w501] -> w489
              tunnel: w488 -> [w497 w500]
              tunnel: [w496 w499] -> w487
              tunnel: FALSE ("Use While Loop?") -> [w494 w498]
              frame "IND560 SERIAL" {
                n344 = Unbundle By Name(w493) -> ("Washer Controls In.Test Fixture Hardware.Weight Scale.Com Options.IND560Scale VISA"=w492:refnum<visa-resource-name>)
                n345 = call "IND560 Serial Tester.vi"("Use While Loop?"=w494, "Error In"=w497, "VISA Input"=w492) -> ("Error Out"=w496:errorcluster, "Net Weight"=w495:dbl)  [unwired: 7 in]
              }
              frame "GSE 350", Default {
                n346 = Unbundle By Name(w503) -> ("Washer Controls In.Test Fixture Hardware.Weight Scale.Com Options.GSE 350"=w502:refnum<visa-resource-name>)
                n347 = call "GSE 350 Main.vi"("Use While Loop?"=w498, "Error In"=w500, "VISA Refnum in"=w502) -> ("Error Out"=w499:errorcluster, "Weight (lb/kg)"=w501:dbl)  [unwired: 6 in, 1 out]
              }
            }
            n348 = local write "Cold Dryer Weigth"(w489) -> ()
            n349 = call <vilib>:"Clear Errors.vi"("error in (no error)"=w487) -> ("error out"=w490:errorcluster)  [unwired: 5 in, 1 out]
          }
          event Value Change {
            n350 = event-data() -> ("NewVal"=w504:T5)  [unwired: 1 in, 5 out]
            n351 = case shown="\"Other\"" w504 {
              frame "D2-Automatic Dryer", Default {
                n352 = property on="Cycles Per Year" class="DigNum (strict)"("Value"=283.0) -> ()  [unwired: 2 in, 2 out]
                n353 = property on="Moisture Reduction Factor" class="DigNum (strict)"("Value"=0.0) -> ()  [unwired: 2 in, 2 out]
                n354 = property on="Field Use Factor" class="DigNum (strict)"("Value"=0.0) -> ()  [unwired: 2 in, 2 out]
              }
              frame "D2-Timer Dryer" {
                n355 = property on="Cycles Per Year" class="DigNum (strict)"("Value"=283.0) -> ()  [unwired: 2 in, 2 out]
                n356 = property on="Moisture Reduction Factor" class="DigNum (strict)"("Value"=55.5) -> ()  [unwired: 2 in, 2 out]
                n357 = property on="Field Use Factor" class="DigNum (strict)"("Value"=1.18) -> ()  [unwired: 2 in, 2 out]
              }
              frame "D1-Automatic Dryer" {
                n358 = property on="Cycles Per Year" class="DigNum (strict)"("Value"=283.0) -> ()  [unwired: 2 in, 2 out]
                n359 = property on="Moisture Reduction Factor" class="DigNum (strict)"("Value"=53.5) -> ()  [unwired: 2 in, 2 out]
                n360 = property on="Field Use Factor" class="DigNum (strict)"("Value"=1.04) -> ()  [unwired: 2 in, 2 out]
              }
              frame "D1-Timer Dryer" {
                n361 = property on="Cycles Per Year" class="DigNum (strict)"("Value"=283.0) -> ()  [unwired: 2 in, 2 out]
                n362 = property on="Moisture Reduction Factor" class="DigNum (strict)"("Value"=53.5) -> ()  [unwired: 2 in, 2 out]
                n363 = property on="Field Use Factor" class="DigNum (strict)"("Value"=1.18) -> ()  [unwired: 2 in, 2 out]
              }
              frame "Other" {
                n364 = property on="Cycles Per Year" class="DigNum (strict)"("Value"=283.0) -> ()  [unwired: 2 in, 2 out]
                n365 = property on="Moisture Reduction Factor" class="DigNum (strict)"("Value"=0.0) -> ()  [unwired: 2 in, 2 out]
                n366 = property on="Field Use Factor" class="DigNum (strict)"("Value"=0.0) -> ()  [unwired: 2 in, 2 out]
              }
            }
            n367 = call <vilib>:"Add State(s) to Queue__jki_lib_state_machine.vi"("State(s) in (\"\")"=w506) -> ("States Out"=w507:string)  [unwired: 14 in]
          }
          event Panel Close? {
            # "Discard the event because we'll close the front panel ourselves in Macro: Exit"
            # "Close Panel button (pressed) Event\n(this executes Macro: Exit to terminate the VI)"
            n368 = event-data() -> ()  [unwired: 1 in, 1 out]
            n369 = call <vilib>:"Add State(s) to Queue__jki_lib_state_machine.vi"("State(s) in Front (\"\")"="Macro: Exit", "State(s) in (\"\")"=w529) -> ("States Out"=w528:string)  [unwired: 13 in]
            n370 = event-data("Discard?"=TRUE) -> ()  [unwired: 1 in, 1 out]
          }
        }
      }
      frame "---------- Core ----------" {
        n371 = call <vilib>:"Add State(s) to Queue__jki_lib_state_machine.vi"("State(s) in (\"\")"=w533) -> ("States Out"=w532:string)  [unwired: 14 in]
      }
      frame Default {
        w543 = 42 items=["No error", "Argument error", "Memory is full", "Out of zone", "End of file", "File already open", "Generic file I/O error", "File not found", "File permission error", "Disk is full", "Duplicate path", "Too many files open", "System feature not enabled", "Resource file not found", "Cannot add resource", "Resource not found", "Image not found", "Image memory error", "Pen does not exist", "Config type invalid", "Config token not found", "Config parse error", "Config memory error", "Bad external code format", "Bad external code offset", "External code not present", "Null window", "Destroy window error", "Null menu", "Print aborted", "Bad print record", "Print driver error", "Windows error during printing", "Memory error during printing", "Print dialog error", "Generic print error", "Invalid device refnum", "Device not found", "Device parameter error", "Device unit error", "Cannot open device", "Device call aborted", "Generic error", "Cancelled by user", "Object ID too low", "Object ID too high", "Object not in heap", "Unknown heap", "Unknown object (invalid DefProc)", "Unknown object (DefProc not in table)", "Message out of range", "Invalid (null) method", "Unknown message", "Manager call not supported", "Bad address", "Network operation in progress", "Network operation timed out", "Connection is busy", "Network attribute not supported", "Network error", "Address in use", "System out of memory", "Connection aborted", "Connection refused", "Not connected", "Already connected", "Connection closed", "Initialization error (interapplication manager)", "Bad occurrence", "Wait on unbound occurrence handler", "Occurrence queue overflow", "Datalog type conflict", "Unused", "Unrecognized type (interapplication manager)", "Memory corrupt", "Failed to make temporary DLL", "Old CIN version", "Drag socket not found", "Failed to load drop-object", "Failed to register OLE object", "Failed to release OLE object", "Format specifier type mismatch", "Unknown format specifier", "Too few format specifiers", "Too many format specifiers", "Scan failed", "Newer CIN version", "Error converting to variant", "Runtime menu error", "Password tampered", "Variant attribute not found", "Incompatible variant data type", "Event data is not available", "Event Store is not present", "Occurrence is not found", "Event Queue is not created", "Event info is not available", "Refnum passed is NULL", "Error retrieving Class GUID", "Error retrieving CoClass GUID", "Error retrieving TypeLib GUID.", "Bad built application magic bytes.", "Specific driver is different from the specific driver associated with the Logical Name.", "There is no session opened to the class driver.", "Max Error", "MAX - Error with config objects", "MAX - Error loading configuration", "MAX - Group not supported"]
        # "Current State"
        # "Handle mistyped state name (developer tool)"
        n372 = Format Into String(format string="Software Exception: Unhandled State \"%s\"." ("message"), error in=w539, w534) -> (resulting string=w542:string, error out=w541:errorcluster)  [unwired: 1 in]
        n373 = call <vilib>:"Error Cluster From Error Code.vi"("show call chain? (False)"=TRUE, "error in (no error)"=w541, "error message (\"\")"=w542, "error code (0)"=w543) -> ("error out"=w540:errorcluster)  [unwired: 5 in]
        n374 = call <vilib>:"Add State(s) to Queue__jki_lib_state_machine.vi"("State(s) in (\"\")"=w538) -> ("States Out"=w537:string)  [unwired: 14 in]
      }
      frame "Initialize Core Data" {
        # "originally closed?"
        # "exe?"
        # "If panel starts closed or is an EXE, then close it when we exit"
        n375 = property class="VI"() -> ("Front Panel.Open"=w553:bool)  [unwired: 2 in, 2 out]
        n376 = property class="App"() -> ("App.Kind"=w552:T28)  [unwired: 2 in, 2 out]
        n377 = control-ref of="Current VI Reference"() -> (w546:refnum<vi>)
        n378 = Not(x=w553) -> (.not. x?=w550:bool)
        n379 = Equal?(x=w552, y=T28."Run Time System" ("Application:Kind")) -> (x = y?=w549:bool)
        n380 = Or(x=w550, y=w549) -> (x .or. y?=w547:bool)
        n381 = Bundle By Name(cluster=w548, "Core.Current VI Reference"=w546, "Core.Close Panel on Exit?"=w547) -> (w554:T31)
        n382 = call <vilib>:"Add State(s) to Queue__jki_lib_state_machine.vi"("State(s) in (\"\")"=w556) -> ("States Out"=w555:string)  [unwired: 14 in]
      }
      frame "Error Handler" {
        # "Unhandled Error -- Display it"
        # "Handle any errors here.\nYou can also output any states to clean-up after errors occur"
        # "Clear error"
        n383 = call <vilib>:"General Error Handler.vi"("error in (no error)"=w561) -> ()  [unwired: 10 in, 5 out]
        n384 = Bundle By Name(cluster=w559, "Error Flag"=TRUE) -> (w558:T31)
        n385 = call <vilib>:"Add State(s) to Queue__jki_lib_state_machine.vi"("State(s) in Front (\"\")"="Macro: Exit", "State(s) in (\"\")"=w564) -> ("States Out"=w563:string)  [unwired: 13 in]
        "Unhandled Error" <- w561
      }
      frame "Exit" {
        n386 = call <vilib>:"Add State(s) to Queue__jki_lib_state_machine.vi"("State(s) in (\"\")"=w569) -> ("States Out"=w568:string)  [unwired: 14 in]
      }
      frame "---------- Data ----------" {
        n387 = call <vilib>:"Add State(s) to Queue__jki_lib_state_machine.vi"("State(s) in (\"\")"=w573) -> ("States Out"=w572:string)  [unwired: 14 in]
      }
      frame "Data: Initialize" {
        w577 = T30 {"Manufacturer-Dish (Array):"=[], "Unit Control-Dish (Array):"=[], "Test Type (Array):"=[], "Cycle Mode-Dish(Array): "=[], "Inlet Temperature (F)-Dish (Array):"=[], "Detergent-Dish (Array):"=[], "Cycle Selection (Array):"=[], "Wash Temperature (Array):"=[], "Rinse Temperature (Array):"=[], "Load Size (Array):"=[], "Water Pressure (PSI) (Array) :"=[], "Ambient RH (Array):"=[], "Supply Voltage (Array):"=[], "Station ID (Array):"=[], "Lab ID (Array):"=[], "TR Number (Array):"=[], "Cold Water Temperature (Fahrenheit) (Array):"=[], "Technician (Array):"=[], "Frequency (Array):"=[], "Build (Array):"=[], "Hot Water Temperature (Fahrenheit) (Array):"=[], "Heating Mode (Array):"=[], "Ambient Temperature (F) (Array):"=[], "Dryer Type (Array):"=[], "Exhaust (Array):"=[], "Drying Cycle (Array):"=[], "Heat Setting (Array):"=[], "Dryness Setting (Array):"=[], "Nominal Load Weigth (lbs) (Array):"=[], "Load Type (Array):"=[]}  # Drop Down Controls
        w580 = T32 {"Current VI Reference"=refnum, "Close Panel on Exit?"=FALSE}  # Core
        w581 = FALSE  # Error Flag
        n388 = local write "Program Tab"(T1."Main" ("Program Tab")) -> ()
        n389 = call <vilib>:"Add State(s) to Queue__jki_lib_state_machine.vi"("State(s) in (\"\")"=w585) -> ("States Out"=w584:string)  [unwired: 14 in]
        n390 = Unbundle By Name("Washer Controls In") -> ("Initialize.Washer In.Appliance Details.Appliance Common.Cycles Per Year"=w575:u32)
        n391 = Bundle("Core"=w580, "Error Flag"=w581, "Washer Controls In"="Washer Controls In", "LV Program"="LV Program", "Filepath In"="Filepath In", "Drop Down Controls"=w577) -> (w583:T31)  [unwired: 1 in]
        n392 = property on="Cycles Per Year" class="DigNum (strict)"("Value"=w575) -> ()  [unwired: 2 in, 2 out]
      }
      frame "Load Configuration" {
        # "This prevents overwriting data that is already good.\n\nLoad the config file...then open the front panel"
        # "Update with correct info"
        n393 = Unbundle By Name(w597) -> ("Washer Controls In.Test Fixture Hardware"=w590:T13, "LV Program"=w594:T9, "Filepath In.General Setup Paths.File Save Configuration Data Path"=w588:path)
        n394 = call "Save File DOE Configuration.vi"("Add/Remove Enum"=T27."Load Standard", "error in (no error)"=w599, "File Save Configuration Data Path"=w588) -> ("error out"=w600:errorcluster, "Full Data Output"=w593:string[][])  [unwired: 6 in, 1 out]
        n395 = call "Save File DOE Extract Configuration Data.vi"("Test Fixture Hardware"=w590, "LV Program"=w594, "Input Config Files"=w593) -> ("Drop Down Core Output"=w596:T33, "Test Fixture Hardware Output"=w595:T13, "Filepath Output"=w587:T10)  [unwired: 6 in]
        n396 = Unbundle By Name(w587) -> ("General Setup Paths.Data Folder Path"=w586:path)
        n397 = Unbundle By Name(w596) -> ("Drop Down Controls"=w591:T30)
        n398 = case shown="Default" w589 {
          tunnel: w597 -> [w606 w611]
          tunnel: w595 -> [_ w610]
          tunnel: [w605 w609] -> w592
          tunnel: w591 -> [w604 w608]
          tunnel: w586 -> [w603 w607]
          frame "Open Front Panel" {
            n399 = Bundle By Name(cluster=w606, "Filepath In.General Setup Paths.Data Folder Path"=w603, "Drop Down Controls"=w604) -> (w605:T31)
          }
          frame Default {
            n400 = Bundle By Name(cluster=w611, "Filepath In.General Setup Paths.Data Folder Path"=w607, "Washer Controls In.Test Fixture Hardware"=w610, "Drop Down Controls"=w608) -> (w609:T31)
          }
        }
        n401 = call <vilib>:"Add State(s) to Queue__jki_lib_state_machine.vi"("State(s) in (\"\")"=w602) -> ("States Out"=w601:string)  [unwired: 14 in]
      }
      frame "Populate Controls" {
        # "Update with correct info"
        n402 = Unbundle By Name(w620) -> ("Drop Down Controls.Manufacturer-Dish (Array):"=w641:string[], "Drop Down Controls.Unit Control-Dish (Array):"=w640:string[], "Drop Down Controls.Test Type (Array):"=w639:string[], "Drop Down Controls.Cycle Mode-Dish(Array):"=w638:string[], "Drop Down Controls.Inlet Temperature (F)-Dish (Array):"=w637:string[], "Drop Down Controls.Detergent-Dish (Array):"=w636:string[], "Drop Down Controls.Cycle Selection (Array):"=w635:string[], "Drop Down Controls.Wash Temperature (Array):"=w634:string[], "Drop Down Controls.Rinse Temperature (Array):"=w633:string[], "Drop Down Controls.Load Size (Array):"=w632:string[], "Drop Down Controls.Water Pressure (PSI) (Array) :"=w631:string[], "Drop Down Controls.Ambient RH (Array):"=w630:string[], "Drop Down Controls.Supply Voltage (Array):"=w629:string[], "Drop Down Controls.Station ID (Array):"=w621:string[], "Drop Down Controls.Lab ID (Array):"=w628:string[], "Drop Down Controls.TR Number (Array):"=w627:string[], "Drop Down Controls.Cold Water Temperature (Fahrenheit) (Array):"=w626:string[], "Drop Down Controls.Technician (Array):"=w625:string[], "Drop Down Controls.Frequency (Array):"=w624:string[], "Drop Down Controls.Build (Array):"=w623:string[], "Drop Down Controls.Hot Water Temperature (Fahrenheit) (Array):"=w622:string[], "Drop Down Controls.Ambient Temperature (F) (Array):"=w619:string[], "Drop Down Controls.Dryer Type (Array):"=w618:string[], "Drop Down Controls.Exhaust (Array):"=w617:string[], "Drop Down Controls.Drying Cycle (Array):"=w616:string[], "Drop Down Controls.Heat Setting (Array):"=w615:string[], "Drop Down Controls.Dryness Setting (Array):"=w614:string[], "Drop Down Controls.Nominal Load Weigth (lbs) (Array):"=w613:string[], "Drop Down Controls.Load Type (Array):"=w612:string[])  [unwired: 1 out]
        n403 = property on="Manufacturer-Dish:" class="CmbBox"("Strings[]"=w641) -> ()  [unwired: 2 in, 2 out]
        n404 = property on="Unit Control-Dish:" class="CmbBox"("Strings[]"=w640) -> ()  [unwired: 2 in, 2 out]
        n405 = property on="Test Type:" class="CmbBox"("Strings[]"=w639) -> ()  [unwired: 2 in, 2 out]
        n406 = property on="Cycle Mode-Dish:" class="CmbBox"("Strings[]"=w638) -> ()  [unwired: 2 in, 2 out]
        n407 = property on="Inlet Temperature-Dish:" class="CmbBox"("Strings[]"=w637) -> ()  [unwired: 2 in, 2 out]
        n408 = property on="Detergent-Dish:" class="CmbBox"("Strings[]"=w636) -> ()  [unwired: 2 in, 2 out]
        n409 = property on="Cycle Selection" class="CmbBox"("Strings[]"=w635) -> ()  [unwired: 2 in, 2 out]
        n410 = property on="Wash Temperature" class="CmbBox"("Strings[]"=w634) -> ()  [unwired: 2 in, 2 out]
        n411 = property on="Rinse Temperature" class="CmbBox"("Strings[]"=w633) -> ()  [unwired: 2 in, 2 out]
        n412 = property on="Load Size" class="CmbBox"("Strings[]"=w632) -> ()  [unwired: 2 in, 2 out]
        n413 = property on="Water Pressure (PSI):" class="CmbBox"("Strings[]"=w631) -> ()  [unwired: 2 in, 2 out]
        n414 = property on="Ambient RH:" class="CmbBox"("Strings[]"=w630) -> ()  [unwired: 2 in, 2 out]
        n415 = property on="Supply Voltage:" class="CmbBox"("Strings[]"=w629) -> ()  [unwired: 2 in, 2 out]
        n416 = property on="Station ID:" class="CmbBox"("Strings[]"=w621) -> ()  [unwired: 2 in, 2 out]
        n417 = property on="Lab ID:" class="CmbBox"("Strings[]"=w628) -> ()  [unwired: 2 in, 2 out]
        n418 = property on="TR Number:" class="CmbBox"("Strings[]"=w627) -> ()  [unwired: 2 in, 2 out]
        n419 = property on="Cold Water Temperature (Fahrenheit)" class="CmbBox"("Strings[]"=w626) -> ()  [unwired: 2 in, 2 out]
        n420 = property on="Technician:" class="CmbBox"("Strings[]"=w625) -> ()  [unwired: 2 in, 2 out]
        n421 = property on="Frequency:" class="CmbBox"("Strings[]"=w624) -> ()  [unwired: 2 in, 2 out]
        n422 = property on="Build:" class="CmbBox"("Strings[]"=w623) -> ()  [unwired: 2 in, 2 out]
        n423 = property on="Hot Water Temperature (Fahrenheit)" class="CmbBox"("Strings[]"=w622) -> ()  [unwired: 2 in, 2 out]
        n424 = property on="Ambient Temperature (F):" class="CmbBox"("Strings[]"=w619) -> ()  [unwired: 2 in, 2 out]
        n425 = property on="Dryer Type:" class="CmbBox"("Strings[]"=w618) -> ()  [unwired: 2 in, 2 out]
        n426 = property on="Exhaust:" class="CmbBox"("Strings[]"=w617) -> ()  [unwired: 2 in, 2 out]
        n427 = property on="Drying Cycle:" class="CmbBox"("Strings[]"=w616) -> ()  [unwired: 2 in, 2 out]
        n428 = property on="Heat Setting:" class="CmbBox"("Strings[]"=w615) -> ()  [unwired: 2 in, 2 out]
        n429 = property on="Dryness Setting:" class="CmbBox"("Strings[]"=w614) -> ()  [unwired: 2 in, 2 out]
        n430 = property on="Nominal Load Weight (lbs):" class="CmbBox"("Strings[]"=w613) -> ()  [unwired: 2 in, 2 out]
        n431 = property on="Load Type:" class="CmbBox"("Strings[]"=w612) -> ()  [unwired: 2 in, 2 out]
        n432 = call <vilib>:"Add State(s) to Queue__jki_lib_state_machine.vi"("State(s) in (\"\")"=w644) -> ("States Out"=w643:string)  [unwired: 14 in]
      }
      frame "Data: Cleanup" {
        n433 = Unbundle By Name(w645) -> ("Core.Current VI Reference"=w648:refnum<vi>)
        n434 = Close Reference(reference=w648, error in (no error)=w647) -> (error out=w646:errorcluster)
        n435 = call <vilib>:"Add State(s) to Queue__jki_lib_state_machine.vi"("State(s) in (\"\")"=w650) -> ("States Out"=w649:string)  [unwired: 14 in]
      }
      frame "---------- UI ----------" {
        n436 = call <vilib>:"Add State(s) to Queue__jki_lib_state_machine.vi"("State(s) in (\"\")"=w654) -> ("States Out"=w653:string)  [unwired: 14 in]
      }
      frame "UI: Initialize" {
        n437 = Unbundle By Name(w664) -> ("Filepath In.General Setup Paths.Tool Base Path"=w658:path)  [unwired: 1 out]
        n438 = Current VI's Path() -> (path=w670:path)
        n439 = call "UTILITY This VIs Path.vi"("path"=w670) -> ("FileVersionInfo Out"=w665:T23)  [unwired: 8 in, 6 out]
        n440 = Format Date/Time String(time format string (%c)="Date_%m_%d_%Y_Time_%H_%M") -> (date/time string=w668:string)  [unwired: 2 out]
        n441 = call "UTILITY IP and Computer Name.vi"() -> ("IP Address"=w666:string, "Computer Name"=w667:string)  [unwired: 10 in]
        n442 = call "Save File General Main File Save Configuration Path.vi"("Error In"=w657, "Tool Base Path"=w658) -> ("Error Out"=w663:errorcluster, "Appliance Previous Run Path"=w660:path, "Calibration File Path"=w661:path, "File Save Configuration Data Path"=w662:path, "DOE Capacity Path"=w659:path)  [unwired: 5 in]
        n443 = Bundle By Name(cluster=w664, "Washer Controls In.Initialize.Washer In.Appliance Details.FileVersionInfo"=w665, "Washer Controls In.Initialize.Washer In.Appliance Details.Appliance Common.Test Date:"=w668, "Washer Controls In.Initialize.Washer In.Appliance Details.Appliance Common.Computer Name:"=w667, "Washer Controls In.Initialize.Washer In.Appliance Details.Appliance Common.IP Address:"=w666, "Filepath In.General Setup Paths.DOE Capacity Path"=w659, "Filepath In.General Setup Paths.File Save Configuration Data Path"=w662, "Filepath In.General Setup Paths.Calibration File Path"=w661, "Filepath In.General Setup Paths.File Save Previous Run Path"=w660) -> (w656:T31)
        n444 = Unbundle By Name(w656) -> ("Filepath In"=w655:T10)
        n445 = local write "Filepath In"(w655) -> ()
        n446 = call <vilib>:"Add State(s) to Queue__jki_lib_state_machine.vi"("State(s) in (\"\")"=w672) -> ("States Out"=w671:string)  [unwired: 14 in]
      }
      frame "UI: Cursor Set" {
        # "Argument"
        # "Set and Unset Cursor Busy.\n(Usage: \"UI: Cursor Set >> Busy|Idle\")"
        n447 = case shown="\"Idle\", Default" w673 {
          tunnel: w675 -> [w680 w682]
          tunnel: [w679 w681] -> w674
          frame "Idle", Default {
            n448 = call <vilib>:"Unset Busy.vi"("error in (no error)"=w680) -> ("error out"=w679:errorcluster)  [unwired: 10 in]
          }
          frame "Busy" {
            n449 = call <vilib>:"Set Busy.vi"("error in (no error)"=w682) -> ("error out"=w681:errorcluster)  [unwired: 9 in, 1 out]
          }
        }
        n450 = call <vilib>:"Add State(s) to Queue__jki_lib_state_machine.vi"("State(s) in (\"\")"=w678) -> ("States Out"=w677:string)  [unwired: 14 in]
      }
      frame "UI: Front Panel State" {
        # "Argument"
        # "Set Front Panel Open or Closed\n(Usage: \"UI: Front Panel State >> Open|Close\")"
        n451 = Unbundle By Name(w685) -> ("Core.Current VI Reference"=w684:refnum<vi>)
        n452 = case shown="\"Open\", Default" w683 {
          tunnel: w687 -> [w693 w706]
          tunnel: [w695 w707] -> w686
          tunnel: w684 -> [w694 w704]
          frame "Open", Default {
            n453 = property class="VI"(reference=w694, error in=w693) -> (reference out=w691:refnum<vi>, error out=w692:errorcluster, "Front Panel.Open"=w690:bool)
            n454 = case shown="False" w690 {
              tunnel: [w698 w701] -> w695
              tunnel: w692 -> [w697 w701]
              tunnel: w691 -> [w696 _]
              frame False {
                n455 = invoke class="VI" method="FP.Open"(reference=w696, error in=w697, "Activate"=TRUE, "State"=T29."Standard") -> (error out=w698:errorcluster)  [unwired: 1 in, 4 out]
              }
              frame True {
              }
            }
          }
          frame "Close" {
            n456 = property class="VI"(reference=w704, error in=w706) -> (reference out=w703:refnum<vi>, error out=w705:errorcluster, "Front Panel.Open"=w702:bool)
            n457 = case shown="True" w702 {
              tunnel: [w708 w711] -> w707
              tunnel: w705 -> [w708 w710]
              tunnel: w703 -> [_ w709]
              frame False {
              }
              frame True {
                n458 = invoke class="VI" method="FP.Close"(reference=w709, error in=w710) -> (error out=w711:errorcluster)  [unwired: 1 in, 2 out]
              }
            }
          }
        }
        n459 = call <vilib>:"Add State(s) to Queue__jki_lib_state_machine.vi"("State(s) in (\"\")"=w689) -> ("States Out"=w688:string)  [unwired: 14 in]
      }
      frame "---------- Macro ----------" {
        n460 = call <vilib>:"Add State(s) to Queue__jki_lib_state_machine.vi"("State(s) in (\"\")"=w715) -> ("States Out"=w714:string)  [unwired: 14 in]
      }
      frame "Macro: Initialize" {
        n461 = property on="OK" class="Bool"("Key Focus"=FALSE) -> ()  [unwired: 2 in, 2 out]
        n462 = local write "Build:"("" ("Dryer Type:")) -> ()
        n463 = call <vilib>:"Add State(s) to Queue__jki_lib_state_machine.vi"("State(s) in Front (\"\")"="Data: Initialize\nInitialize Core Data\nUI: Initialize", "State(s) in (\"\")"=w722) -> ("States Out"=w721:string)  [unwired: 13 in]
      }
      frame "Macro: Exit" {
        n464 = Unbundle By Name(w729) -> ("Core.Close Panel on Exit?"=w723:bool)
        n465 = Select(t="UI: Front Panel State >> Close", s=w723, f="") -> (s? t:f=w726:string)
        n466 = call <vilib>:"Add State(s) to Queue__jki_lib_state_machine.vi"("State(s) in (\"\")"=w726, "State(s) at Back (\"\")"="Data: Cleanup\nExit") -> ("States Out"=w724:string)  [unwired: 13 in]
        n467 = call <vilib>:"Add State(s) to Queue__jki_lib_state_machine.vi"("State(s) in Front (\"\")"=w724, "State(s) in (\"\")"=w732) -> ("States Out"=w731:string)  [unwired: 13 in]
      }
      frame "---------- New Category ----------" {
        n468 = call <vilib>:"Add State(s) to Queue__jki_lib_state_machine.vi"("State(s) in (\"\")"=w736) -> ("States Out"=w735:string)  [unwired: 14 in]
      }
      frame "Get Main Info" {
        n469 = Equal?(x="Station ID:", y="Select Room/Stall") -> (x = y?=w739:bool)
        n470 = case shown="False" w739 {
          tunnel: "Station ID:" -> [w761 _]
          tunnel: [w761 w762] -> w737
          frame False {
          }
          frame True {
            w762 = ""
            n471 = local write "Station ID:"(w762) -> ()
          }
        }
        n472 = Bundle By Name(cluster=w756, "Washer Controls In.Initialize.Washer In.Appliance Details.Appliance Common.TR Number:"="TR Number:", "Washer Controls In.Initialize.Washer In.Appliance Details.Appliance Common.Lab ID:"="Lab ID:", "Washer Controls In.Initialize.Washer In.Appliance Details.Appliance Common.Model Number:"="Model:", "Washer Controls In.Initialize.Washer In.Appliance Details.Appliance Common.Serial Number:"="Serial Number:", "Washer Controls In.Initialize.Washer In.Display Data (RLT).Serial Number Display"="Serial Number:", "Washer Controls In.Initialize.Washer In.Appliance Details.Appliance Common.Station ID:"=w737, "Washer Controls In.Initialize.Washer In.Display Data (RLT).Station Label Display"=w737, "Washer Controls In.Initialize.Washer In.Appliance Details.Appliance Common.Engineer:"="Engineer:", "Washer Controls In.Initialize.Washer In.Appliance Details.Appliance Common.Technician:"="Technician:", "Washer Controls In.Initialize.Washer In.Appliance Details.Appliance Common.Water Pressure (PSI):"="Water Pressure (PSI):", "Washer Controls In.Initialize.Washer In.Appliance Details.Appliance Common.Ambient RH:"="Ambient RH:", "Washer Controls In.Initialize.Washer In.Appliance Details.Appliance Common.Ambient Temperature (F):"="Ambient Temperature (F):", "Washer Controls In.Initialize.Washer In.Appliance Details.Appliance Common.Voltage:"="Supply Voltage:", "Washer Controls In.Initialize.Washer In.Appliance Details.Appliance Common.Frequency:"="Frequency:", "Washer Controls In.Initialize.Washer In.Appliance Details.Appliance Common.Build:"="Build:", "Washer Controls In.Initialize.Washer In.Appliance Details.Appliance Common.Comments:"="Comments:", "Washer Controls In.Initialize.Washer In.Appliance Details.Appliance Common.Test Type:"="Test Type:", "Washer Controls In.Initialize.Washer In.Appliance Details.Appliance Common.Load Run #:"="Load Run #:") -> (w758:T31)
        n473 = call <vilib>:"Add State(s) to Queue__jki_lib_state_machine.vi"("State(s) in (\"\")"=w757) -> ("States Out"=w760:string)  [unwired: 14 in]
      }
      frame "Check Contents" {
        # "If all of the data fields have information go ahead and generate the filename"
        n474 = Unbundle By Name(w775) -> ("Washer Controls In.Initialize.Washer In.Appliance Details.Appliance Common.TR Number:"=w773:string, "Washer Controls In.Initialize.Washer In.Appliance Details.Appliance Common.Lab ID:"=w772:string, "Washer Controls In.Initialize.Washer In.Appliance Details.Appliance Common.Serial Number:"=w771:string, "Washer Controls In.Initialize.Washer In.Appliance Details.Appliance Common.Station ID:"=w770:string, "Washer Controls In.Initialize.Washer In.Appliance Details.Dryer.Dryer Initial IMC Data.Measured IMC In Range?"=w767:bool, "LV Program"=w763:T9)
        n475 = Build Array(w773, w772, w771, w770) -> (w769:string[])
        n476 = for {
          tunnel: w769 -> [w787] mode=indexing
          tunnel: [w786] -> w768 mode=indexing
          n477 = String Length(string=w787) -> (length=w788:i32)
          n478 = Greater Than 0?(x=w788) -> (x > 0?=w786:bool)
        }
        n479 = And Array Elements(Boolean array=w768) -> (logical AND=w765:bool)
        n480 = case shown="Default" w763 {
          tunnel: w767 -> [_ w783]
          tunnel: ["You Must ENTER the following:\n1. TR Number                 \n2. Lab ID                          \n3. Serial Number            \n4. Station ID                    " ("message") "You Must ENTER the following:\n1. TR Number \n2. Lab ID \n3. Serial Number\n4. Station ID\n5. Initial Moisure Content Info                    " ("message")] -> w766
          tunnel: w765 -> [w780 w784]
          tunnel: [w780 w782] -> w764
          frame Default {
          }
          frame "Dryer" {
            n481 = And(x=w784, y=w783) -> (x .and. y?=w782:bool)
          }
        }
        n482 = case shown="True" w764 {
          tunnel: ["" w792] -> w776
          tunnel: w775 -> [w790 w794]
          tunnel: [w790 w794] -> w774
          tunnel: w763 -> [_ w793]
          tunnel: w766 -> [w789 _]
          frame False {
            n483 = One Button Dialog(message=w789) -> ()  [unwired: 1 in, 1 out]
          }
          frame True {
            n484 = case shown="\"Refrigeration\"" w793 {
              tunnel: ["Get Washer Info\nGenerate Filename\nGenerate Header Data" "Get Dish Info\nGenerate Filename\nGenerate Header Data" "Get HEWH Info\nGenerate Filename\nGenerate Header Data" "Get Dryer Info\nGenerate Filename\nGenerate Header Data" "Get Refrigeration\nGenerate Filename\nGenerate Header Data"] -> w792
              frame "DOE Stand", "Portable Stand", Default {
              }
              frame "Dishwasher Kitchen" {
              }
              frame "HEWH", "PRAT", "HEWH RLT" {
              }
              frame "Dryer" {
              }
              frame "Refrigeration" {
              }
            }
          }
        }
        n485 = call <vilib>:"Add State(s) to Queue__jki_lib_state_machine.vi"("State(s) in Front (\"\")"=w776, "State(s) in (\"\")"=w779) -> ("States Out"=w778:string)  [unwired: 13 in]
      }
      frame "Get Dish Info" {
        n486 = Unbundle By Name(w808) -> ("LV Program"=w807:T9)
        n487 = case shown="\"Dishwasher Kitchen\"" w807 {
          tunnel: w808 -> [w813 w822 w823 w824]
          tunnel: [w813 w821 w823 w824] -> w810
          tunnel: "Manufacturer-Dish:" -> [_ w820 _ _]
          tunnel: "Unit Control-Dish:" -> [_ w819 _ _]
          tunnel: "Cycle Mode-Dish:" -> [_ w818 _ _]
          tunnel: "Inlet Temperature-Dish:" -> [_ w817 _ _]
          tunnel: "Detergent-Dish:" -> [_ w816 _ _]
          tunnel: "Auto Cup Weight (gm):" -> [_ w815 _ _]
          tunnel: "Open Cup Weight (gm):" -> [_ w814 _ _]
          frame "DOE Stand", "Portable Stand", Default {
          }
          frame "Dishwasher Kitchen" {
            n488 = Bundle By Name(cluster=w822, "Washer Controls In.Initialize.Washer In.Appliance Details.Dishwasher Info.Manufacturer-Dish:"=w820, "Washer Controls In.Initialize.Washer In.Appliance Details.Dishwasher Info.Unit Control-Dish:"=w819, "Washer Controls In.Initialize.Washer In.Appliance Details.Dishwasher Info.Cycle Mode-Dish:"=w818, "Washer Controls In.Initialize.Washer In.Appliance Details.Dishwasher Info.Inlet Temperature-Dish:"=w817, "Washer Controls In.Initialize.Washer In.Appliance Details.Dishwasher Info.Detergent-Dish:"=w816, "Washer Controls In.Initialize.Washer In.Appliance Details.Dishwasher Info.Auto Cup Weight (gm):"=w815, "Washer Controls In.Initialize.Washer In.Appliance Details.Dishwasher Info.Open Cup Weight (gm):"=w814) -> (w821:T31)
          }
          frame "HEWH", "PRAT", "HEWH RLT" {
          }
          frame "Dryer" {
          }
        }
        n489 = call <vilib>:"Add State(s) to Queue__jki_lib_state_machine.vi"("State(s) in (\"\")"=w809) -> ("States Out"=w812:string)  [unwired: 14 in]
      }
      frame "Get Washer Info" {
        n490 = Unbundle By Name(w838) -> ("LV Program"=w837:T9)
        n491 = case shown="\"DOE Stand\", \"Portable Stand\", Default" w837 {
          tunnel: w838 -> [w856 w857 w858 w859]
          tunnel: [w855 w857 w858 w859] -> w840
          tunnel: "Model Family" -> [w854 _ _ _]
          tunnel: "Program Name" -> [w853 _ _ _]
          tunnel: "Cycle Selection" -> [w852 _ _ _]
          tunnel: "Wash Temperature" -> [w851 _ _ _]
          tunnel: "Rinse Temperature" -> [w850 _ _ _]
          tunnel: "Load Size" -> [w849 _ _ _]
          tunnel: "Hot Water Temperature (Fahrenheit)" -> [w848 _ _ _]
          tunnel: "Cold Water Temperature (Fahrenheit)" -> [w847 _ _ _]
          tunnel: "Capacity (cu.ft)" -> [w846 _ _ _]
          tunnel: "Initial Cloth Weight:" -> [w845 _ _ _]
          tunnel: "Cloth Lot:" -> [w844 _ _ _]
          tunnel: "Unit Type Display" -> [w843 _ _ _]
          frame "DOE Stand", "Portable Stand", Default {
            n492 = Bundle By Name(cluster=w856, "Washer Controls In.Initialize.Washer In.Appliance Details.Washer Info.Model Family:"=w854, "Washer Controls In.Initialize.Washer In.Appliance Details.Washer Info.Program Name:"=w853, "Washer Controls In.Initialize.Washer In.Appliance Details.Washer Info.Cycle Selection:"=w852, "Washer Controls In.Initialize.Washer In.Appliance Details.Washer Info.Wash Temperature:"=w851, "Washer Controls In.Initialize.Washer In.Appliance Details.Washer Info.Rinse Temperature:"=w850, "Washer Controls In.Initialize.Washer In.Appliance Details.Washer Info.Load Size:"=w849, "Washer Controls In.Initialize.Washer In.Appliance Details.Washer Info.Hot Water Temperature (Fahrenheit):"=w848, "Washer Controls In.Initialize.Washer In.Appliance Details.Washer Info.Cold Water Temperature (Fahrenheit):"=w847, "Washer Controls In.Initialize.Washer In.Appliance Details.Washer Info.Capacity (cu.ft):"=w846, "Washer Controls In.Initialize.Washer In.Appliance Details.Washer Info.Initial Cloth Weight:"=w845, "Washer Controls In.Initialize.Washer In.Appliance Details.Washer Info.Cloth Lot:"=w844, "Washer Controls In.Initialize.Washer In.Display Data (RLT).Unit Type Display"=w843) -> (w855:T31)
          }
          frame "Dishwasher Kitchen" {
          }
          frame "HEWH", "PRAT", "HEWH RLT" {
          }
          frame "Dryer" {
          }
        }
        n493 = call <vilib>:"Add State(s) to Queue__jki_lib_state_machine.vi"("State(s) in (\"\")"=w839) -> ("States Out"=w842:string)  [unwired: 14 in]
      }
      frame "Get HEWH Info" {
        n494 = Unbundle By Name(w862) -> ("LV Program"=w861:T9)
        n495 = case shown="\"HEWH\", \"PRAT\", \"HEWH RLT\"" w861 {
          tunnel: w862 -> [w867 w868 w871 w872]
          tunnel: [w867 w868 w870 w872] -> w864
          tunnel: "Heating Mode" -> [_ _ w869 _]
          frame "DOE Stand", "Portable Stand", Default {
          }
          frame "Dishwasher Kitchen" {
          }
          frame "HEWH", "PRAT", "HEWH RLT" {
            n496 = Bundle By Name(cluster=w871, "Washer Controls In.Initialize.Washer In.Appliance Details.Water Heater.Heating Mode:"=w869) -> (w870:T31)
          }
          frame "Dryer" {
          }
        }
        n497 = call <vilib>:"Add State(s) to Queue__jki_lib_state_machine.vi"("State(s) in (\"\")"=w863) -> ("States Out"=w866:string)  [unwired: 14 in]
      }
      frame "Get Dryer Info" {
        n498 = Unbundle By Name(w888) -> ("LV Program"=w887:T9)
        n499 = case shown="\"Dryer\"" w887 {
          tunnel: w888 -> [w893 w894 w895 w911]
          tunnel: [w893 w894 w895 w910] -> w890
          tunnel: "Heat Setting:" -> [_ _ _ w909]
          tunnel: "Washer Water Temperature (60 ± 5°F):" -> [_ _ _ w908]
          tunnel: "Water Hardness (PPM):" -> [_ _ _ w907]
          tunnel: "Dryness Setting:" -> [_ _ _ w906]
          tunnel: "Dryer Type:" -> [_ _ _ w905]
          tunnel: "Exhaust:" -> [_ _ _ w904]
          tunnel: "Drying Cycle:" -> [_ _ _ w903]
          tunnel: "Cold Dryer Weigth" -> [_ _ _ w902]
          tunnel: "Load Type:" -> [_ _ _ w901]
          tunnel: "Nominal Load Weight (lbs):" -> [_ _ _ w900]
          tunnel: "Cycles Per Year" -> [_ _ _ w899]
          tunnel: "Moisture Reduction Factor" -> [_ _ _ w898]
          tunnel: "Field Use Factor" -> [_ _ _ w897]
          tunnel: "Energy Standard" -> [_ _ _ w896]
          frame "DOE Stand", "Portable Stand", Default {
          }
          frame "Dishwasher Kitchen" {
          }
          frame "HEWH", "PRAT", "HEWH RLT" {
          }
          frame "Dryer" {
            n500 = Bundle By Name(cluster=w911, "Washer Controls In.Initialize.Washer In.Appliance Details.Dryer.Dryer Initial IMC Data.Energy Standard"=w896, "Washer Controls In.Initialize.Washer In.Appliance Details.Dryer.Heat Setting:"=w909, "Washer Controls In.Initialize.Washer In.Appliance Details.Dryer.Washer Water Temperature (60 ± 5°F):"=w908, "Washer Controls In.Initialize.Washer In.Appliance Details.Dryer.Water Hardness (PPM):"=w907, "Washer Controls In.Initialize.Washer In.Appliance Details.Dryer.Dryness Setting:"=w906, "Washer Controls In.Initialize.Washer In.Appliance Details.Dryer.Dryer Type:"=w905, "Washer Controls In.Initialize.Washer In.Appliance Details.Dryer.Exhaust:"=w904, "Washer Controls In.Initialize.Washer In.Appliance Details.Dryer.Drying Cycle:"=w903, "Washer Controls In.Initialize.Washer In.Appliance Details.Dryer.Dryer Initial IMC Data.Empty Dryer Cold Weigth"=w902, "Washer Controls In.Initialize.Washer In.Appliance Details.Dryer.Load Type:"=w901, "Washer Controls In.Initialize.Washer In.Appliance Details.Dryer.Nominal Load Weight"=w900, "Washer Controls In.Initialize.Washer In.Appliance Details.Appliance Common.Cycles Per Year"=w899, "Washer Controls In.Initialize.Washer In.Appliance Details.Dryer.Dryer Initial IMC Data.Moisture Reduction Factor"=w898, "Washer Controls In.Initialize.Washer In.Appliance Details.Dryer.Dryer Initial IMC Data.Field Use Factor"=w897) -> (w910:T31)
          }
        }
        n501 = call <vilib>:"Add State(s) to Queue__jki_lib_state_machine.vi"("State(s) in (\"\")"=w889) -> ("States Out"=w892:string)  [unwired: 14 in]
      }
      frame "Get Refrigeration" {
        n502 = Unbundle By Name(w913) -> ("LV Program"=w912:T9)
        n503 = case shown="\"Refrigeration\"" w912 {
          tunnel: w913 -> [w918 w919 w920 w921 w922]
          tunnel: [w918 w919 w920 w921 w922] -> w915
          frame "DOE Stand", "Portable Stand", Default {
          }
          frame "Dishwasher Kitchen" {
          }
          frame "HEWH", "PRAT", "HEWH RLT" {
          }
          frame "Dryer" {
          }
          frame "Refrigeration" {
            # "Get Refrigeration specifics later"
          }
        }
        n504 = call <vilib>:"Add State(s) to Queue__jki_lib_state_machine.vi"("State(s) in (\"\")"=w914) -> ("States Out"=w917:string)  [unwired: 14 in]
      }
      frame "Generate Filename" {
        n505 = Unbundle By Name(w930) -> ("LV Program"=w928:T9, "Filepath In"=w929:T10, "Washer Controls In.Initialize.Washer In"=w927:T21)
        n506 = call "Save File Create Filename and Directories.vi"("LV Program"=w928, "Error In"=w924, "Initialize.Washer In"=w927, "File Paths In"=w929) -> ("Error Out"=w923:errorcluster, "Initialize.Washer Out"=w925:T21, "File Paths Out"=w926:T10)  [unwired: 5 in]
        n507 = Bundle By Name(cluster=w930, "Filepath In"=w926, "Washer Controls In.Initialize.Washer In"=w925) -> (w931:T31)
        n508 = call <vilib>:"Add State(s) to Queue__jki_lib_state_machine.vi"("State(s) in (\"\")"=w933) -> ("States Out"=w932:string)  [unwired: 14 in]
      }
      frame "Generate Header Data" {
        # "Check to make sure everything is\ncalibrated If its not, display a message\nto the user"
        n509 = Unbundle By Name(w942) -> ("Washer Controls In.Initialize.Washer In.Appliance Details"=w938:T22, "LV Program"=w937:T9, "Filepath In.General Setup Paths.Calibration File Path"=w936:path)
        n510 = call "Save File DOE Create Header File.vi"("Error In"=w935, "Calibration File Path"=w936, "LV Program"=w937, "Appliance Details"=w938) -> ("Error Out"=w934:errorcluster, "File Initialization Array"=w940:string[][])  [unwired: 6 in]
        n511 = Bundle By Name(cluster=w942, "Washer Controls In.Initialize.Washer In.Appliance Details.File Name Output Array"=w940) -> (w941:T31)
        n512 = call <vilib>:"Add State(s) to Queue__jki_lib_state_machine.vi"("State(s) in Front (\"\")"="Save Appliance Details" ("State(s) in Front (\"\")"), "State(s) in (\"\")"=w944) -> ("States Out"=w943:string)  [unwired: 13 in]
      }
      frame "Save Appliance Details" {
        n513 = Unbundle By Name(w948) -> ("Filepath In"=w947:T10, "Washer Controls In.Initialize.Washer In.Appliance Details"=w951:T22, "Filepath In.General Setup Paths.File Save Previous Run Path"=w950:path)
        n514 = local write "Filepath In"(w947) -> ()
        n515 = call "Save File DOE Save Previous Input Data.vi"("State"=enum16{"Write", "Read"}."Write", "error in (no error)"=w946, "Appliance Previous Run Path"=w950, "Appliance Details"=w951) -> ("error out"=w945:errorcluster)  [unwired: 6 in, 1 out]
        n516 = call <vilib>:"Add State(s) to Queue__jki_lib_state_machine.vi"("State(s) in Front (\"\")"="Macro: Exit" ("State(s) in Front (\"\")"), "State(s) in (\"\")"=w954) -> ("States Out"=w953:string)  [unwired: 13 in]
      }
    }
    n517 = case shown="True" "Debug" {
      tunnel: w19 -> [w30 w33]
      tunnel: [w30 w32] -> w18
      tunnel: w17 -> [_ w31]
      frame False {
      }
      frame True {
        n518 = Build Array (concatenate)(w33, w31) -> (w32:string[])
        "States" <- w32
      }
    }
  }
  "error out" <- w9
  n519 = Unbundle By Name(w6) -> ("Washer Controls In"=→"Washer Controls Out":T12, "Filepath In"=→"Filepath Out":T10)
